vi "1D_Plotter_MATLAB.vi"(1 "Job Directory":path) -> (2 "Saved Automatically?":bool, 3 "gnuplotScript":string, 4 "Plot data file":path)   [LabVIEW 2022 SP3]
uses:
  Data plotting/MATLAB/Plot Style.ctl
  gnuplotScriptComponents/minAndMax.ctl
  gnuplotScriptComponents/AutoManualNumber.ctl
  gnuplotScriptComponents/ticsAndGrids.ctl
  gnuplotScriptComponents/tics.ctl
  gnuplotScriptComponents/grids.ctl
  Error bar Type.ctl
  Data plotting/MATLAB/MATLAB_Mode.ctl
  Results_plotter_Global.vi
  Globals/Constants_global.vi
  Data plotting/subVIs/Plot_Values_Global.vi
panel:
  in  "Tab Control":T1(tab)
  in  "Show Save Option?":bool
  in  "Font Size":string="10"
  in  "MainTitleFontSize":string="12"
  in  "Horizontal/Vertical plot ratio":dbl=1.0 min=0.1 max=10.0 format="%.2f"
  in  "Auto":bool=TRUE
  in  "Open in Acrobat":bool=TRUE
  in  "Stl File":u16(ring)
  in  "Location Y limits":string="-2000;2000"
  in  "Location X limits":string="-2000;2000"
  in  "Plot Location?":bool
  in  "Z Limits Auto":bool=TRUE
  in  "Location Z limits":string="-2000;2000"
  in  "Y Limits Auto":bool=TRUE
  in  "X Limits Auto":bool=TRUE
  in  "Only Show Plots with ALL Series":bool
  in  "nRows":u8=3 min=1
  in  "nCols":u8=3 min=1
  in  "Swop Series and Plots":bool
  in  "Legend Title":string
  out "Number of Figures":i32
  in  "View Angle":string="-20;39"
  in  "lRefArrowSize":string="2"
  in  "lRefArrowColor":string="k"
  in  "lRefArrowComponents":string="300;0;0"
  in  "lRefArrowBaseCoord":string="0;0;0"
  in  "lRefPointSize":string="20"
  in  "lRefPointColor":string="y"
  in  "lRefPointCoord":string="0;0;0"
  in  "fAxisLabelYright":string
  out "Output file":path
  out "Saved Files":path[](array[path])
  in  "Reduce Individual Plot Title Lengths if too long":bool=TRUE
  in  "Show Channels with range of Values?":bool
  in  "ManualPlotTitles":string[](array[string])
  in  "Individual Plot Titles":bool=TRUE
  in  "Page Title Pre Block":string
  in  "Page Title Post Block":string
  in  "Values to include in Page Title":i32[](listbox)
  out "Final Title":string
  out "Plot Titles":string[](array[string])
  in  "Plot Legends Manual":string[](array[string])
  in  "Plotstyles":T2[](array[typedef])=[{"Color"="r", "LStyle"="solid", "LWidth"="0.5", "Marker"="o", "Marker size"="4.0", "Fit?"=FALSE, "Right Y?"=FALSE}, {"Color"="g", "LStyle"="solid", "LWidth"="0.5", "Marker"="+", "Marker size"="4.0", "Fit?"=FALSE, "Right Y?"=FALSE}, {"Color"="b", "LStyle"="solid", "LWidth"="0.5", "Marker"="*", "Marker size"="4.0", "Fit?"=FALSE, "Right Y?"=FALSE}, {"Color"="k", "LStyle"="solid", "LWidth"="0.5", "Marker"=".", "Marker size"="4.0", "Fit?"=FALSE, "Right Y?"=FALSE}, {"Color"="c", "LStyle"="solid", "LWidth"="0.5", "Marker"="x", "Marker size"="4.0", "Fit?"=FALSE, "Right Y?"=FALSE}, {"Color"="m", "LStyle"="solid", "LWidth"="0.5", "Marker"="s", "Marker size"="4.0", "Fit?"=FALSE, "Right Y?"=FALSE}, {"Color"="y", "LStyle"="solid", "LWidth"="0.5", "Marker"="d", "Marker size"="4.0", "Fit?"=FALSE, "Right Y?"=FALSE}, {"Color"="r", "LStyle"="--", "LWidth"="0.5", "Marker"="^", "Marker size"="4.0", "Fit?"=FALSE, "Right Y?"=FALSE}, {"Color"="g", "LStyle"="--", "LWidth"="0.5", "Marker"="v", "Marker size"="4.0", "Fit?"=FALSE, "Right Y?"=FALSE}, {"Color"="b", "LStyle"="--", "LWidth"="0.5", "Marker"="p", "Marker size"="4.0", "Fit?"=FALSE, "Right Y?"=FALSE}, {"Color"="k", "LStyle"="--", "LWidth"="0.5", "Marker"="h", "Marker size"="4.0", "Fit?"=FALSE, "Right Y?"=FALSE}, {"Color"="c", "LStyle"="--", "LWidth"="0.5", "Marker"="x", "Marker size"="4.0", "Fit?"=FALSE, "Right Y?"=FALSE}, {"Color"="m", "LStyle"="--", "LWidth"="0.5", "Marker"=">", "Marker size"="4.0", "Fit?"=FALSE, "Right Y?"=FALSE}] caption="Plot Style"
  out "Plot Legends Auto":string[](array[string])
  out "No of Series supplied":i32
  in  "Plot Legends":bool=TRUE
  in  "Error Bar Type":T3=enum."Standard Error"
  in  "2nd Y Axis":enum8{"Lin", "Log"}(ring)
  in  "Y/R tics And Grids":T4={"tics"={"ticMin"=0.0, "ticStep"=5.0, "ticMax"=0.0, "minorDivsPerMajor"=2, "ticSpacing"=enum."Approx n Tics (rounded)", "ticPosition"=enum."Inside, no mirror"}, "Grids"={"Gridlines"=enum."No grids", "Zeroaxis"=enum."No zero axis"}, "Mapping"=enum."Lin"}
  in  "X/Theta tics And Grids":T4={"tics"={"ticMin"=0.0, "ticStep"=5.0, "ticMax"=0.0, "minorDivsPerMajor"=2, "ticSpacing"=enum."Approx n Tics (rounded)", "ticPosition"=enum."Inside, no mirror"}, "Grids"={"Gridlines"=enum."Major grid", "Zeroaxis"=enum."No zero axis"}, "Mapping"=enum."Lin"}
  in  "PlotType":enum32{"XY", "Time"}(tab)
  in  "yAxisBounds":T7={"Min"={"Auto"=TRUE, "Value"=0.0}, "Max"={"Auto"=TRUE, "Value"=0.0}}
  in  "xAxisBounds":T7={"Min"={"Auto"=TRUE, "Value"=0.0}, "Max"={"Auto"=TRUE, "Value"=0.0}}
  in  "Set bounds using XY Plot \non Results file plotter":bool
  out "Time format?":bool
  in  "Time/Date Format":string(combo)="%I:%M %p\\n%d-%b-%y"
  in  "Select Time Zone":u32(ring)=142 items=["Abbreviation (Time Zone Name)", "A (Alpha Time Zone)", "ACDT (Australian Central Daylight Time  CDT ‚Äì Central Daylight Time CDST ‚Äì Central Daylight Savings Time)", "ACST (Australian Central Standard Time  CST ‚Äì Central Standard Time)", "ACT (Acre Time)", "ACT (Australian Central Time)", "ACWST (Australian Central Western Standard Time)", "ADT (Arabia Daylight Time  AST ‚Äì Arabia Summer Time)", "ADT (Atlantic Daylight Time  ADST ‚Äì Atlantic Daylight Saving Time AST ‚Äì Atlantic Summer Time  HAA ‚Äì Heure Avancv©e de l'Atlantique (French))", "AEDT (Australian Eastern Daylight Time  EDT ‚Äì Eastern Daylight Time EDST ‚Äì Eastern Daylight Saving Time)", "AEST (Australian Eastern Standard Time  EST ‚Äì Eastern Standard Time AET ‚Äì Australian Eastern Time)", "AET (Australian Eastern Time)", "AFT (Afghanistan Time)", "AKDT (Alaska Daylight Time  ADST ‚Äì Alaska Daylight Saving Time)", "AKST (Alaska Standard Time  AT ‚Äì Alaska Time)", "ALMT (Alma-Ata Time)", "AMST (Amazon Summer Time)", "AMST (Armenia Summer Time  AMDT ‚Äì Armenia Daylight Time)", "AMT (Amazon Time)", "AMT (Armenia Time)", "ANAST (Anadyr Summer Time)", "ANAT (Anadyr Time)", "AQTT (Aqtobe Time)", "ART (Argentina Time)", "AST (Arabia Standard Time  AST ‚Äì Arabic Standard Time AST ‚Äì Al Manamah Standard Time)", "AST (Atlantic Standard Time  AT ‚Äì Atlantic Time  AST ‚Äì Tiempo Estv°ndar del Atlv°ntico (Spanish) HNA ‚Äì Heure Normale de l'Atlantique (French))", "AT (Atlantic Time)", "AWDT (Australian Western Daylight Time  WDT ‚Äì Western Daylight Time WST ‚Äì Western Summer Time)", "AWST (Australian Western Standard Time  WST ‚Äì Western Standard Time WAT ‚Äì Western Australia Time)", "AZOST (Azores Summer Time  AZODT ‚Äì Azores Daylight Time)", "AZOT (Azores Time  AZOST ‚Äì Azores Standard Time)", "AZST (Azerbaijan Summer Time)", "AZT (Azerbaijan Time)", "AoE (Anywhere on Earth)", "B (Bravo Time Zone)", "BNT (Brunei Darussalam Time  BDT ‚Äì Brunei Time)", "BOT (Bolivia Time)", "BRST (Brasv?lia Summer Time  BST ‚Äì Brazil Summer Time BST ‚Äì Brazilian Summer Time)", "BRT (Brasv?lia Time  BT ‚Äì Brazil Time BT ‚Äì Brazilian Time)", "BST (Bangladesh Standard Time)", "BST (Bougainville Standard Time)", "BST (British Summer Time  BDT ‚Äì British Daylight Time BDST ‚Äì British Daylight Saving Time)", "BTT (Bhutan Time)", "C (Charlie Time Zone)", "CAST (Casey Time)", "CAT (Central Africa Time)", "CCT (Cocos Islands Time)", "CDT (Central Daylight Time  CDST ‚Äì Central Daylight Saving Time NACDT ‚Äì North American Central Daylight Time  HAC ‚Äì Heure Avancv©e du Centre (French))", "CDT (Cuba Daylight Time)", "CEST (Central European Summer Time  CEDT ‚Äì Central European Daylight Time ECST ‚Äì European Central Summer Time  MESZ ‚Äì Mitteleuropv§ische Sommerzeit (German))", "CET (Central European Time  ECT ‚Äì European Central Time CET ‚Äì Central Europe Time  MEZ ‚Äì Mitteleuropv§ische Zeit (German))", "CHADT (Chatham Island Daylight Time  CDT ‚Äì Chatham Daylight Time)", "CHAST (Chatham Island Standard Time)", "CHOST (Choibalsan Summer Time  CHODT ‚Äì Choibalsan Daylight Time CHODST ‚Äì Choibalsan Daylight Saving Time)", "CHOST (Choibalsan Summer Time)", "CHOT (Choibalsan Time)", "CHUT (Chuuk Time)", "CIDST (Cayman Islands Daylight Saving Time)", "CIST (Cayman Islands Standard Time  CIT ‚Äì Cayman Islands Time)", "CKT (Cook Island Time)", "CLST (Chile Summer Time  CLDT ‚Äì Chile Daylight Time)", "CLT (Chile Standard Time  CT ‚Äì Chile Time CLST ‚Äì Chile Standard Time)", "COT (Colombia Time)", "CST (Central Standard Time  CT ‚Äì Central Time NACST ‚Äì North American Central Standard Time  CST ‚Äì Tiempo Central Estv°ndar (Spanish) HNC ‚Äì Heure Normale du Centre (French))", "CST (China Standard Time)", "CST (Cuba Standard Time)", "CT (Central Time)", "CVT (Cape Verde Time)", "CXT (Christmas Island Time)", "ChST (Chamorro Standard Time  GST ‚Äì Guam Standard Time)", "D (Delta Time Zone)", "DAVT (Davis Time)", "DDUT (Dumont-d'Urville Time)", "E (Echo Time Zone)", "EASST (Easter Island Summer Time  EADT ‚Äì Easter Island Daylight Time)", "EAST (Easter Island Standard Time)", "EAT (Eastern Africa Time  EAT ‚Äì East Africa Time)", "ECT (Ecuador Time)", "EDT (Eastern Daylight Time  EDST ‚Äì Eastern Daylight Savings Time NAEDT ‚Äì North American Eastern Daylight Time  HAE ‚Äì Heure Avancv©e de l'Est (French) EDT ‚Äì Tiempo de verano del Este (Spanish))", "EEST (Eastern European Summer Time  EEDT ‚Äì Eastern European Daylight Time  OESZ ‚Äì Osteuropv§ische Sommerzeit (German))", "EET (Eastern European Time  OEZ ‚Äì Osteuropv§ische Zeit (German))", "EGST (Eastern Greenland Summer Time  EGST ‚Äì East Greenland Summer Time)", "EGT (East Greenland Time  EGT ‚Äì Eastern Greenland Time)", "EST (Eastern Standard Time  ET ‚Äì Eastern Time  NAEST ‚Äì North American Eastern Standard Time  ET ‚Äì Tiempo del Este (Spanish) HNE ‚Äì Heure Normale de l'Est (French))", "ET (Eastern Time)", "F (Foxtrot Time Zone)", "FET (Further-Eastern European Time)", "FJST (Fiji Summer Time  FJDT ‚Äì Fiji Daylight Time)", "FJT (Fiji Time)", "FKST (Falkland Islands Summer Time  FKDT ‚Äì Falkland Island Daylight Time)", "FKT (Falkland Island Time  FKST ‚Äì Falkland Island Standard Time)", "FNT (Fernando de Noronha Time)", "G (Golf Time Zone)", "GALT (Galapagos Time)", "GAMT (Gambier Time  GAMT ‚Äì Gambier Islands Time)", "GET (Georgia Standard Time)", "GFT (French Guiana Time)", "GILT (Gilbert Island Time)", "GMT (Greenwich Mean Time  \"‚Äì Coordinated Universal Time GT ‚Äì Greenwich Time)", "GST (Gulf Standard Time)", "GST (South Georgia Time)", "GYT (Guyana Time)", "H (Hotel Time Zone)", "HADT (Hawaii-Aleutian Daylight Time  HDT ‚Äì Hawaii Daylight Time)", "HAST (Hawaii-Aleutian Standard Time  HST ‚Äì Hawaii Standard Time)", "HKT (Hong Kong Time)", "HOVST (Hovd Summer Time  HOVDT ‚Äì Hovd Daylight Time HOVDST ‚Äì Hovd Daylight Saving Time)", "HOVST (Hovd Summer Time)", "HOVT (Hovd Time)", "I (India Time Zone)", "ICT (Indochina Time)", "IDT (Israel Daylight Time)", "IOT (Indian Chagos Time)", "IRDT (Iran Daylight Time  IRST ‚Äì Iran Summer Time IDT ‚Äì Iran Daylight Time)", "IRKST (Irkutsk Summer Time)", "IRKT (Irkutsk Time)", "IRST (Iran Standard Time  IT ‚Äì Iran Time)", "IST (India Standard Time  IT ‚Äì India Time IST ‚Äì Indian Standard Time)", "IST (Irish Standard Time  IST ‚Äì Irish Summer Time)", "IST (Israel Standard Time)", "JST (Japan Standard Time)", "K (Kilo Time Zone)", "KGT (Kyrgyzstan Time)", "KOST (Kosrae Time)", "KRAST (Krasnoyarsk Summer Time)", "KRAT (Krasnoyarsk Time)", "KST (Korea Standard Time  KST ‚Äì Korean Standard Time KT ‚Äì Korea Time)", "KUYT (Kuybyshev Time  SAMST ‚Äì Samara Summer Time)", "L (Lima Time Zone)", "LHDT (Lord Howe Daylight Time)", "LHST (Lord Howe Standard Time)", "LINT (Line Islands Time)", "M (Mike Time Zone)", "MAGST (Magadan Summer Time  MAGST ‚Äì Magadan Island Summer Time)", "MAGT (Magadan Time  MAGT ‚Äì Magadan Island Time)", "MART (Marquesas Time)", "MAWT (Mawson Time)", "MDT (Mountain Daylight Time  MDST ‚Äì Mountain Daylight Saving Time NAMDT ‚Äì North American Mountain Daylight Time  HAR ‚Äì Heure Avancv©e des Rocheuses (French))", "MHT (Marshall Islands Time)", "MMT (Myanmar Time)", "MSD (Moscow Daylight Time  Moscow Summer Time)", "MSK (Moscow Standard Time  MCK ‚Äì Moscow Time)", "MST (Mountain Standard Time  MT ‚Äì Mountain Time NAMST ‚Äì North American Mountain Standard Time  HNR ‚Äì Heure Normale des Rocheuses (French))", "MT (Mountain Time)", "MUT (Mauritius Time)", "MVT (Maldives Time)", "MYT (Malaysia Time  MST ‚Äì Malaysian Standard Time)", "N (November Time Zone)", "NCT (New Caledonia Time)", "NDT (Newfoundland Daylight Time  HAT ‚Äì Heure Avancv©e de Terre-Neuve (French))", "NFT (Norfolk Time  NFT ‚Äì Norfolk Island Time)", "NOVST (Novosibirsk Summer Time  OMSST ‚Äì Omsk Summer Time)", "NOVT (Novosibirsk Time  OMST ‚Äì Omsk Standard Time)", "NPT (Nepal Time)", "NRT (Nauru Time)", "NST (Newfoundland Standard Time  HNT ‚Äì Heure Normale de Terre-Neuve (French))", "NUT (Niue Time)", "NZDT (New Zealand Daylight Time)", "NZST (New Zealand Standard Time)", "O (Oscar Time Zone)", "OMSST (Omsk Summer Time  NOVST ‚Äì Novosibirsk Summer Time)", "OMST (Omsk Standard Time  OMST ‚Äì Omsk Time NOVT ‚Äì Novosibirsk Time)", "ORAT (Oral Time)", "P (Papa Time Zone)", "PDT (Pacific Daylight Time  PDST ‚Äì Pacific Daylight Saving Time NAPDT ‚Äì North American Pacific Daylight Time  HAP ‚Äì Heure Avancv©e du Pacifique (French))", "PET (Peru Time)", "PETST (Kamchatka Summer Time)", "PETT (Kamchatka Time  PETT ‚Äì Petropavlovsk-Kamchatski Time)", "PGT (Papua New Guinea Time)", "PHOT (Phoenix Island Time)", "PHT (Philippine Time  PST ‚Äì Philippine Standard Time)", "PKT (Pakistan Standard Time  PKT ‚Äì Pakistan Time)", "PMDT (Pierre & Miquelon Daylight Time)", "PMST (Pierre & Miquelon Standard Time)", "PONT (Pohnpei Standard Time)", "PST (Pacific Standard Time  PT ‚Äì Pacific Time NAPST ‚Äì North American Pacific Standard Time  PT ‚Äì Tiempo del Pacv?fico (Spanish) HNP ‚Äì Heure Normale du Pacifique (French))", "PST (Pitcairn Standard Time)", "PT (Pacific Time)", "PWT (Palau Time)", "PYST (Paraguay Summer Time)", "PYT (Paraguay Time)", "PYT (Pyongyang Time  PYST ‚Äì Pyongyang Standard Time)", "PYT (Pyongyang Time)", "Q (Quebec Time Zone)", "QYZT (Qyzylorda Time)", "R (Romeo Time Zone)", "RET (Reunion Time)", "ROTT (Rothera Time)", "S (Sierra Time Zone)", "SAKT (Sakhalin Time)", "SAMT (Samara Time  SAMT ‚Äì Samara Standard Time)", "SAST (South Africa Standard Time  SAST ‚Äì South African Standard Time)", "SBT (Solomon Islands Time  SBT ‚Äì Solomon Island Time)", "SCT (Seychelles Time)", "SGT (Singapore Time  SST ‚Äì Singapore Standard Time)", "SRET (Srednekolymsk Time)", "SRT (Suriname Time)", "SST (Samoa Standard Time)", "SYOT (Syowa Time)", "T (Tango Time Zone)", "TAHT (Tahiti Time)", "TFT (French Southern and Antarctic Time  KIT ‚Äì Kerguelen (Islands) Time)", "TJT (Tajikistan Time)", "TKT (Tokelau Time)", "TLT (East Timor Time)", "TMT (Turkmenistan Time)", "TOT (Tonga Time)", "TVT (Tuvalu Time)", "U (Uniform Time Zone)", "ULAST (Ulaanbaatar Summer Time  ULAST ‚Äì Ulan Bator Summer Time)", "ULAST (Ulaanbaatar Summer Time)", "ULAT (Ulaanbaatar Time  ULAT ‚Äì Ulan Bator Time)", "ULAT (Ulaanbaatar Time)", "UTC (Coordinated Universal Time)", "UYST (Uruguay Summer Time)", "UYT (Uruguay Time)", "UZT (Uzbekistan Time)", "V (Victor Time Zone)", "VET (Venezuelan Standard Time  HLV ‚Äì Hora Legal de Venezuela (Spanish))", "VLAST (Vladivostok Summer Time)", "VLAT (Vladivostok Time)", "VOST (Vostok Time)", "VUT (Vanuatu Time  EFATE ‚Äì Efate Time)", "W (Whiskey Time Zone)", "WAKT (Wake Time)", "WARST (Western Argentine Summer Time)", "WAST (West Africa Summer Time)", "WAT (West Africa Time)", "WEST (Western European Summer Time  WEDT ‚Äì Western European Daylight Time  WESZ ‚Äì Westeuropv§ische Sommerzeit (German))", "WET (Western European Time  GMT ‚Äì Greenwich Mean Time  WEZ ‚Äì Westeuropv§ische Zeit (German))", "WFT (Wallis and Futuna Time)", "WGST (Western Greenland Summer Time  WGST ‚Äì West Greenland Summer Time)", "WGT (West Greenland Time  WGT ‚Äì Western Greenland Time)", "WIB (Western Indonesian Time  WIB ‚Äì Waktu Indonesia Barat)", "WIT (Eastern Indonesian Time  WIT ‚Äì Waktu Indonesia Timur)", "WITA (Central Indonesian Time  WITA ‚Äì Waktu Indonesia Tengah)", "WST (West Samoa Time  ST ‚Äì Samoa Time)", "WST (Western Sahara Summer Time)", "WT (Western Sahara Standard Time  WT ‚Äì Western Sahara Time)", "X (X-ray Time Zone)", "Y (Yankee Time Zone)", "YAKST (Yakutsk Summer Time)", "YAKT (Yakutsk Time)", "YAPT (Yap Time)", "YEKST (Yekaterinburg Summer Time)", "YEKT (Yekaterinburg Time)", "Z (Zulu Time Zone)"]
  out "Time Format String":string="%I:%M %p\\n%d-%b-%y"
  out "Formatted date/time string":string="05:00 PM\\n21-Jan-16"
  out "TZ Shift (hrs)":string="UTC-7.00"
  out "ILocationRotations":string
  out "AuditTrail":string[](array[string])
  out "Desired Legends":string[][](array[string])
  out "Table":string[][](table)
  in  "Put Coeff\nin Results file":bool
  in  "Fit type":T9(ring)=enum."Gauss Vert"
  out "Coeff":string[][](array[string])
  out "subarray":string[](array[string])
  out "Plot Array":i32[][](array[numeric])
  in  "stl file String":string="MAGIC_London_Southbank_0_deg.stl"
  out "Array":path[](array[path])
  out "stl Limits":sgl[][](array[numeric])
  out "Legend Location":string
  out "No of Series":i32
  out "Dont show axis label":bool
  out "Duplicate Plot":bool
  out "Multi_Plot":bool
  out "Y labels":bool[](array[boolean])
  out "X Labels":bool[](array[boolean])
  out "Plot Array initial":i32[][](array[numeric])
  out "Plot Folder":string[](array[string])
  out "Max Min array":dbl[][][](array[numeric])
  out "Error Bars":bool[][](array[boolean])
  out "Y Names":string[](array[string])
  out "X Names":string[](array[string])
  out "X Pos":dbl[](array[numeric])
  out "Y Pos":dbl[](array[numeric])
  out "Z Pos":dbl[](array[numeric])
  # "Rows/ Columns/ Series from: controls not wired- just a thought for explicit control of what goes where...?"
  # "Location Plot"
  # "Overall Page Title"
  # "There are as many graphs as there are titles (from Selector 2)...."
  # "Plot Styles"
  # "Each graph contains plots from Selector 1..."
  # "X"
  # "Y"
  # "Shows the numbered line colours and point styles available- well it would, if it didn't disappear every time I update from the repository..!"
  # "You have to save the plot for this to work"
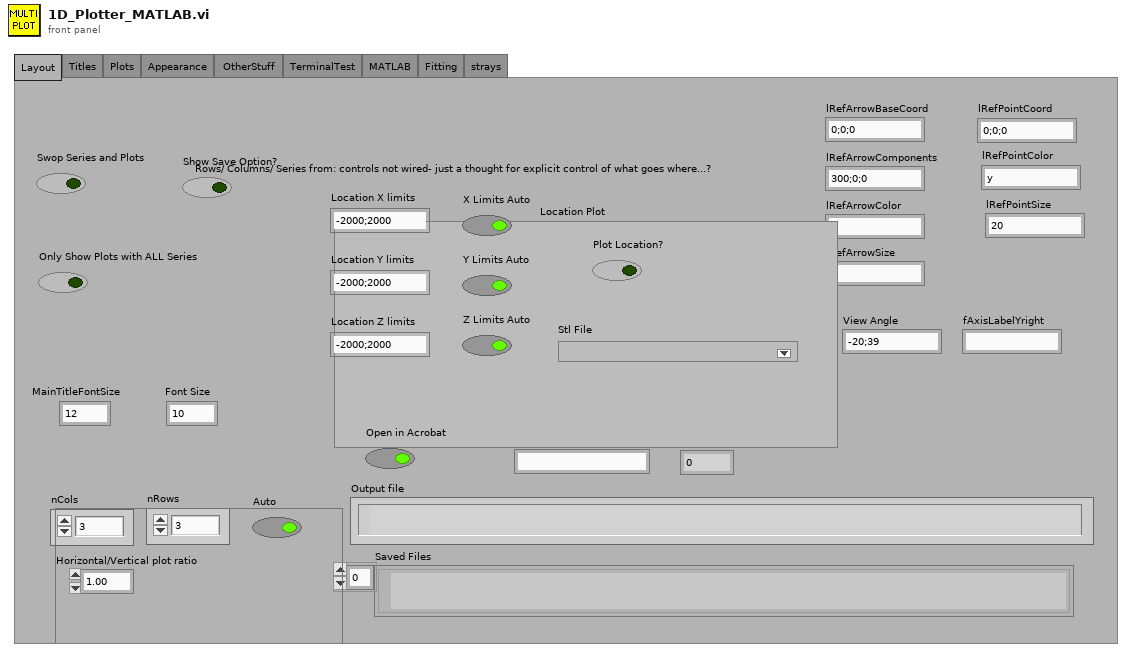
[diagram p1: front panel]
types:
  T1 = enum32{"Layout", "Titles", "Plots", "Appearance", "OtherStuff ", "TerminalTest", "MATLAB", "Fitting", "strays"}
  T2 = typedef "Plot Style.ctl" = cluster{"Color":string, "LStyle":string, "LWidth":string, "Marker":string, "Marker size":string, "Fit?":bool, "Right Y?":bool}
  T3 = typedef "Error bar Type.ctl" = enum16{"None", "Standard Error", "Separate upper and lower"}
  T4 = typedef "ticsAndGrids.ctl" = cluster{"tics":T5, "Grids":T6, "Mapping":enum8{"Lin", "Log"}}
  T5 = typedef "tics.ctl" = cluster{"ticMin":dbl, "ticStep":dbl, "ticMax":dbl, "minorDivsPerMajor":i32, "ticSpacing":enum16{"Auto Tics", "Fixed spacing", "Fixed Minimum and Spacing", "Start, Spacing and Maximum", "Approx n Tics (rounded)"}, "ticPosition":enum16{"Inside, no mirror", "Inside, mirrored", "Outside, no mirror", "Outside, mirrored", "Invisible"}}
  T6 = typedef "grids.ctl" = cluster{"Gridlines":enum16{"No grids", "Major grid", "Minor grid", "Major and Minor"}, "Zeroaxis":enum16{"No zero axis", "Show zero axis"}}
  T7 = typedef "minAndMax.ctl" = cluster{"Min":T8, "Max":T8}
  T8 = typedef "AutoManualNumber.ctl" = cluster{"Auto":bool, "Value":dbl}
  T9 = enum16{"None", "Linear", "2nd Poly", "3rd Poly", "4th Poly", "Gauss Lat", "Gauss Vert", "Guass glc"}
  T10 = enum16{"No grids", "Major grid", "Minor grid", "Major and Minor"}
  T11 = typedef "MATLAB_Mode.ctl" = enum16{"1D Plotter", "2D Plotter", "LP Plotter", "7HP UVW"}
  T12 = typedef "RFP_Plot_Metadata.ctl" = cluster{"Row Number":i32[], "Error Bars":T13, "X Label":string, "Y Label":string, "Blanks NaNs":i32[]}
  T13 = typedef "Error_bars_index.ctl" = cluster{"Upper":i32, "Lower":i32, "St Error":i32}
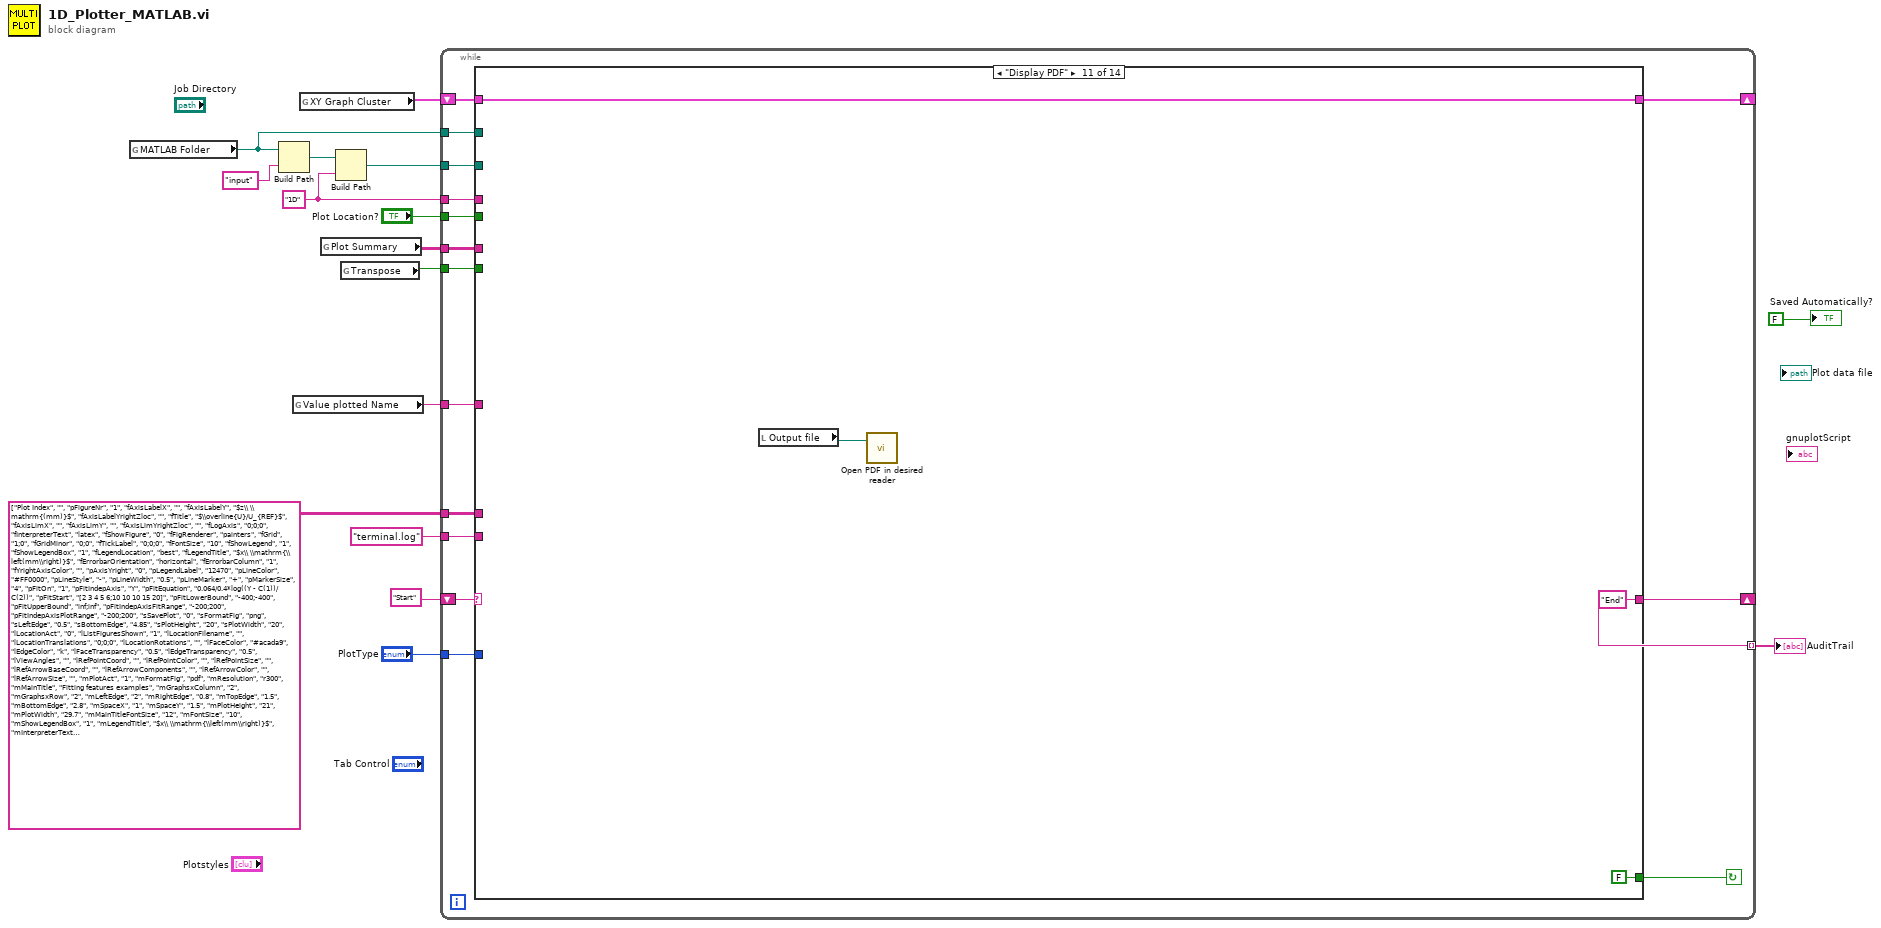
[diagram p0: block diagram]
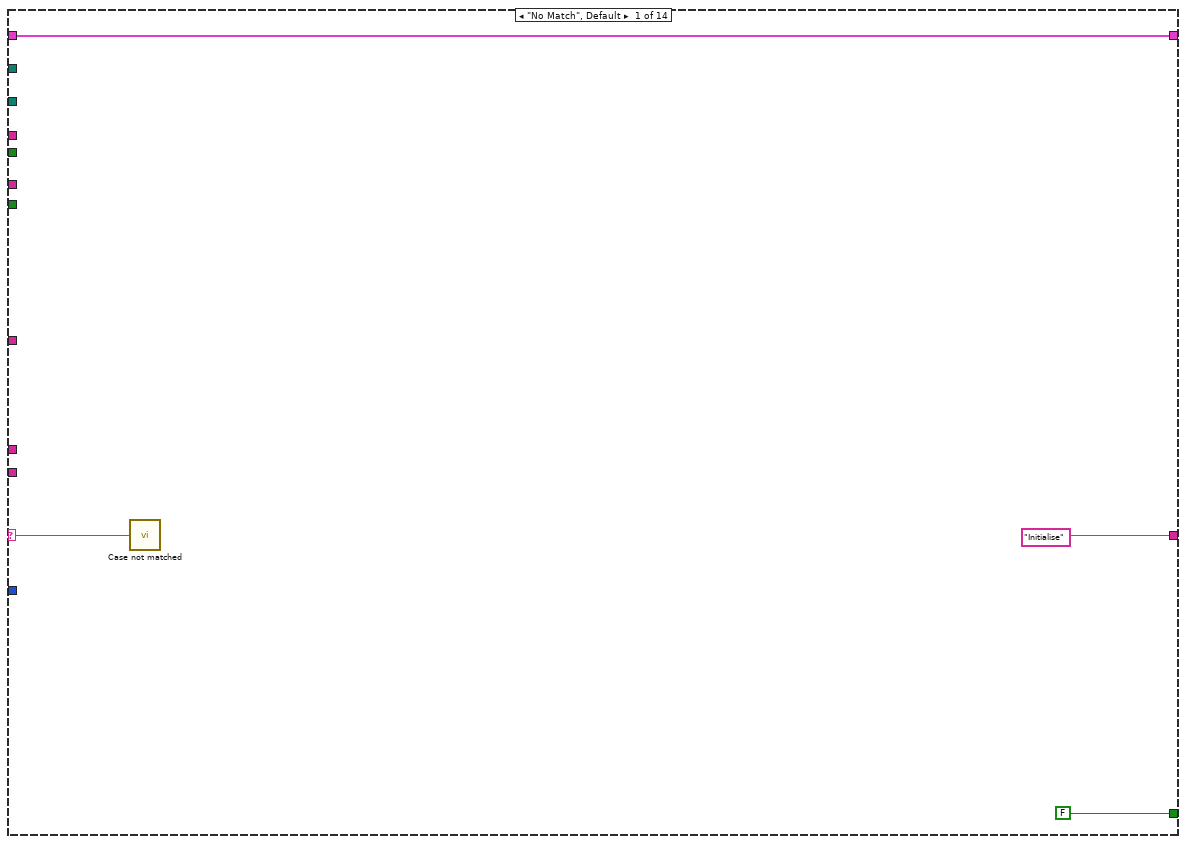
[diagram p2: hidden frame]
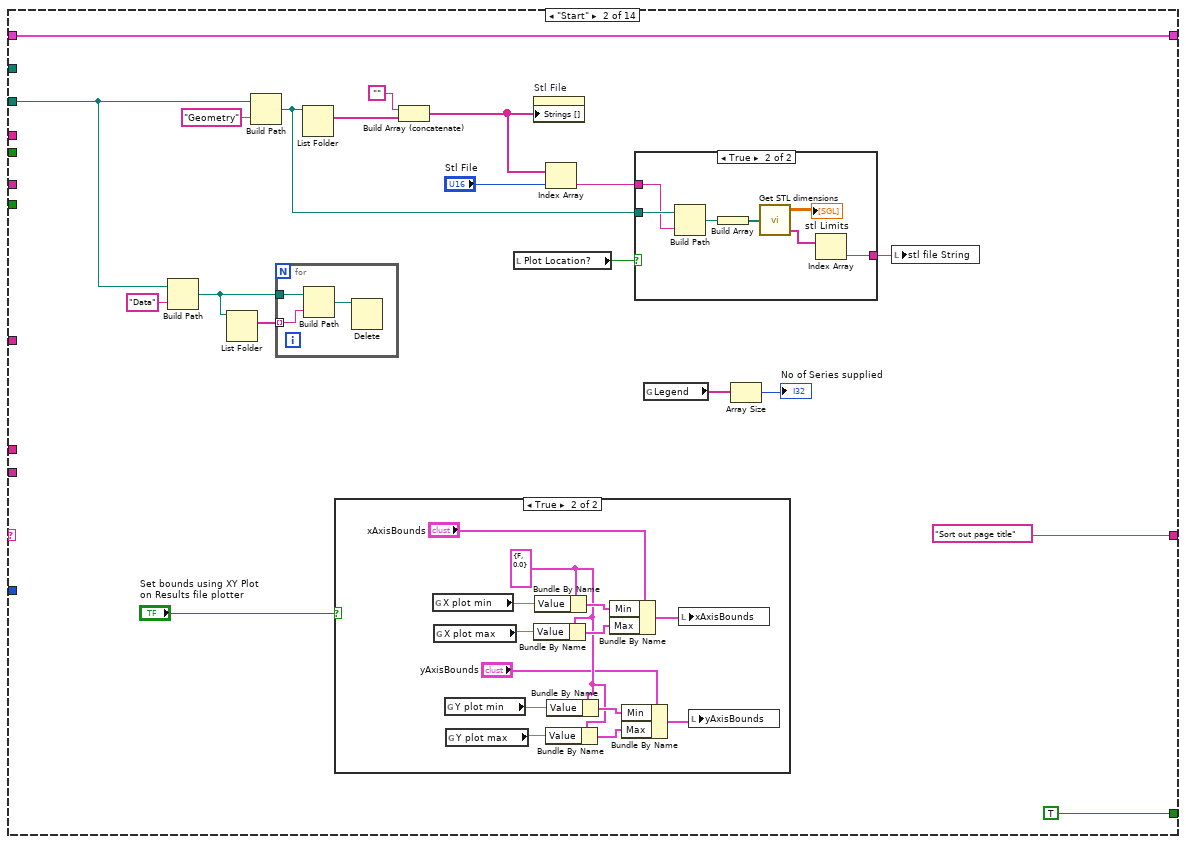
[diagram p3: hidden frame]
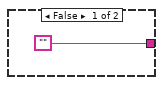
[diagram p4: hidden frame]
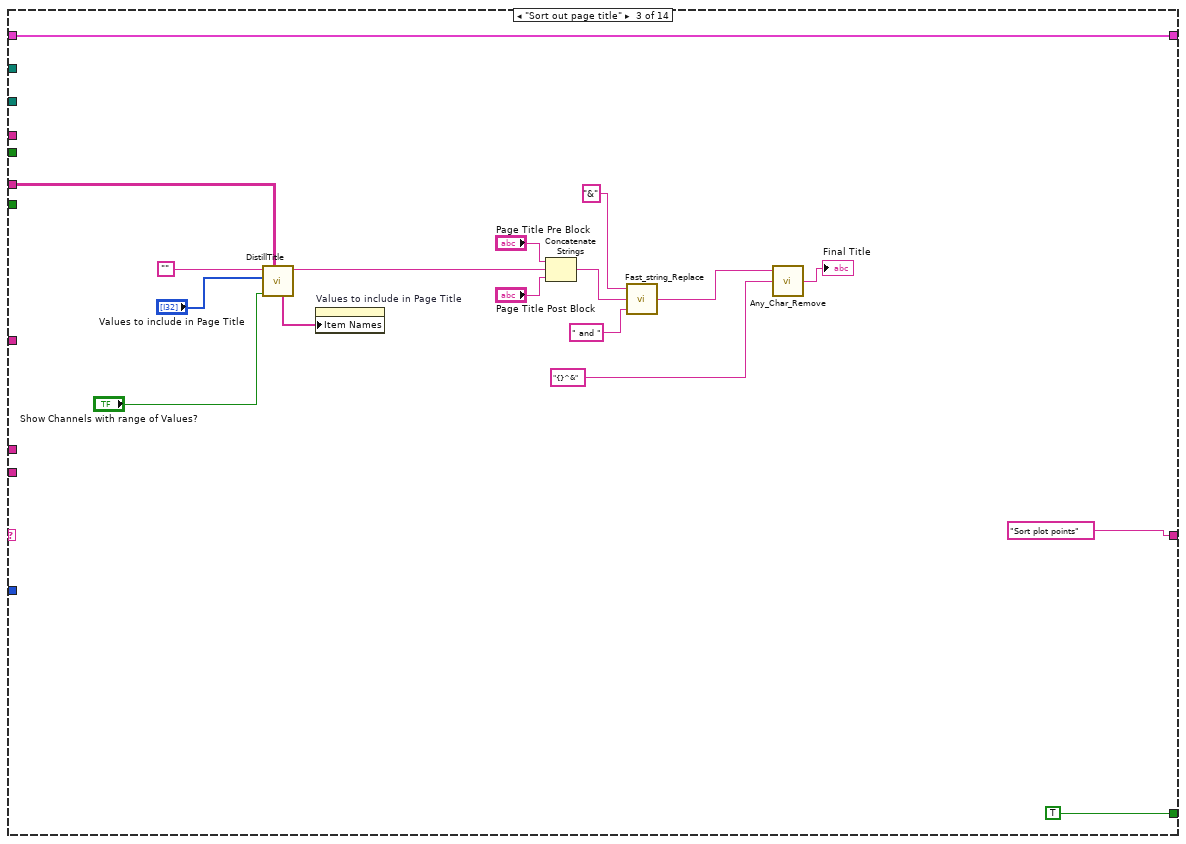
[diagram p6: hidden frame]
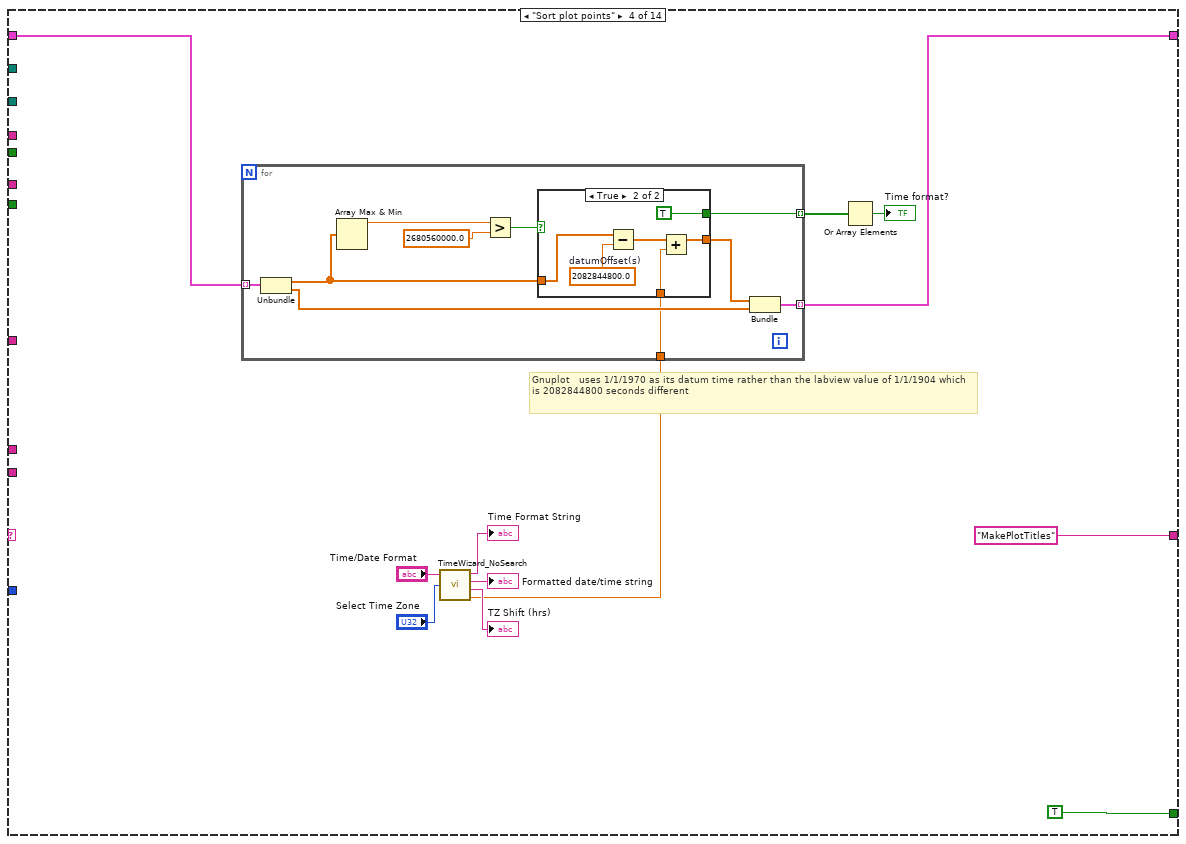
[diagram p7: hidden frame]
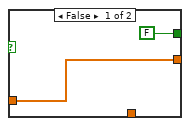
[diagram p8: hidden frame]
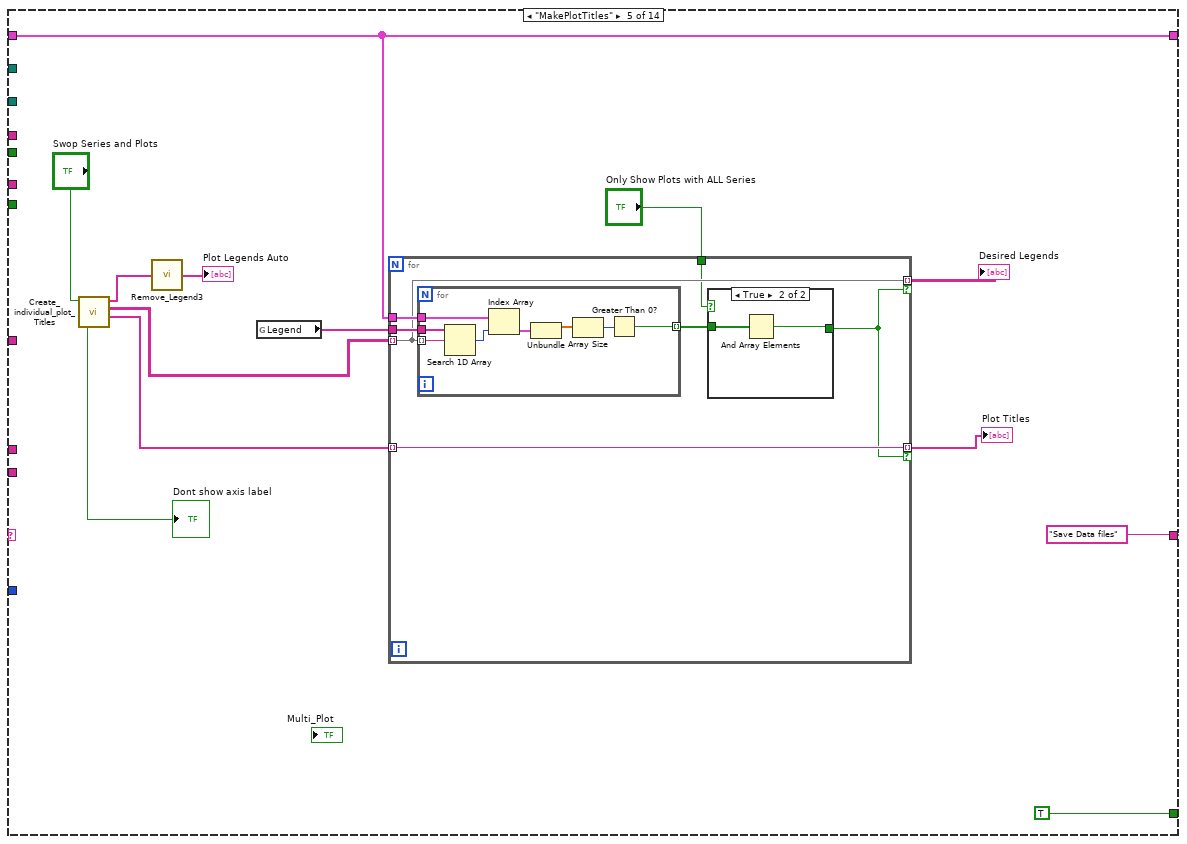
[diagram p9: hidden frame]
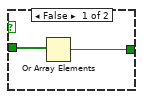
[diagram p10: hidden frame]
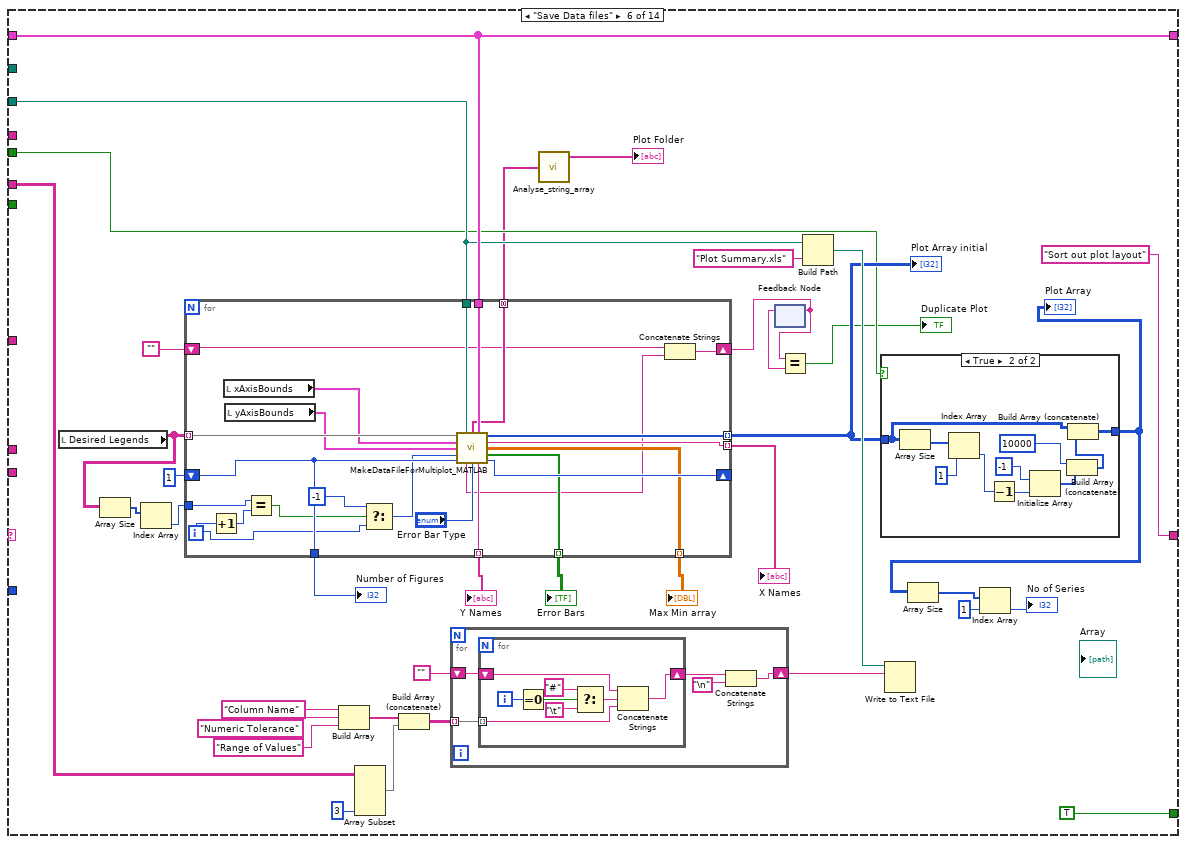
[diagram p11: hidden frame]
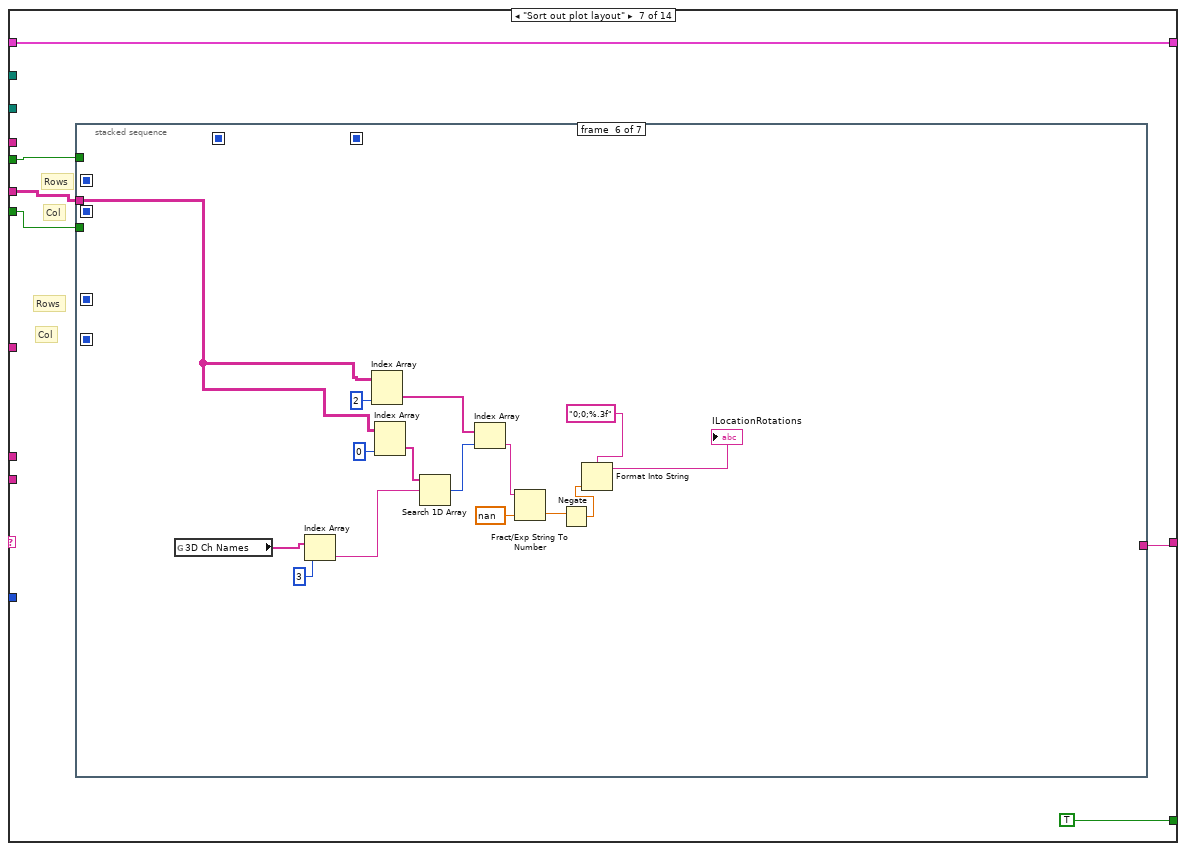
[diagram p13: hidden frame]
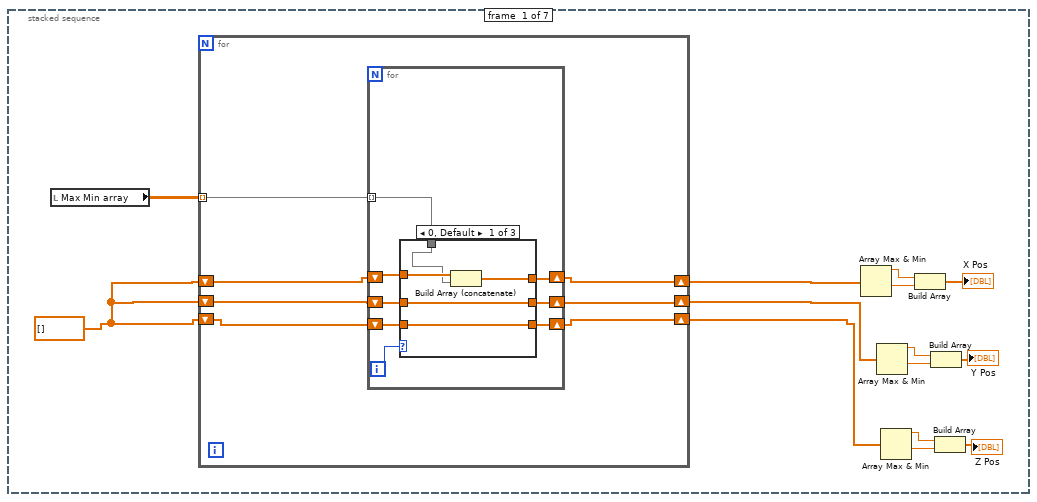
[diagram p14: hidden frame]
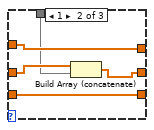
[diagram p15: hidden frame]
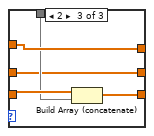
[diagram p16: hidden frame]
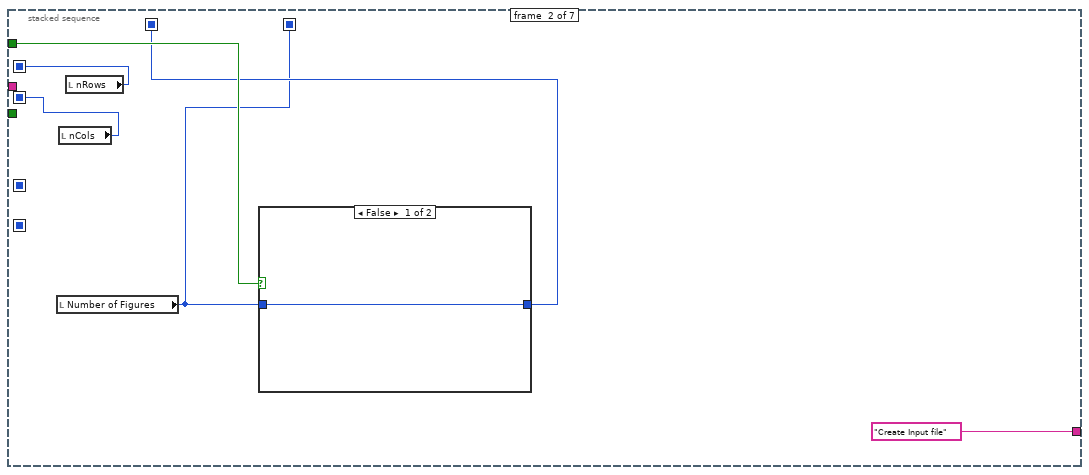
[diagram p17: hidden frame]
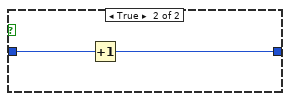
[diagram p18: hidden frame]
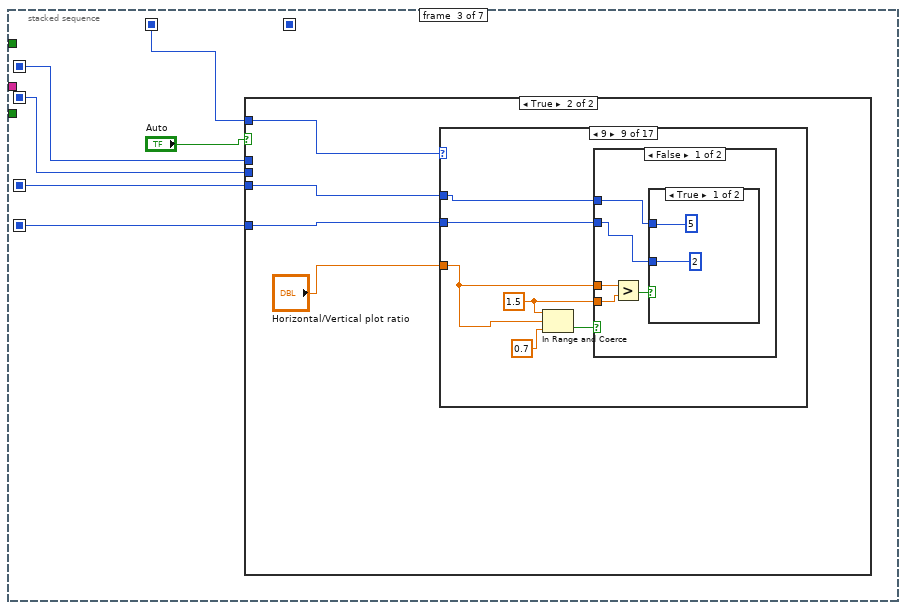
[diagram p19: hidden frame]
diagram:
  w1 = "1D" ("name or relative path")
  n1 = global read "Constants_global.vi" "MATLAB Folder"() -> (w2:path)
  n2 = Build Path(base path=w2, name or relative path="input") -> (appended path=w8:path)
  n3 = global read "Results_plotter_Global.vi" "Value plotted Name"() -> (w14:string)
  n4 = global read "Plot_Values_Global.vi" "XY Graph Cluster"() -> (w3:cluster{dbl[], dbl[]}[])
  n5 = global read "Results_plotter_Global.vi" "Plot Summary"() -> (w15:string[][])
  n6 = Build Path(base path=w8, name or relative path=w1) -> (appended path=w7:path)
  n7 = global read "Results_plotter_Global.vi" "Transpose"() -> (w4:bool)
  n8 = while {
    shift-left: "Start" -> [w30]
    shift-right: [w23] -> _
    tunnel: w15 -> [w29]
    tunnel: w14 -> [w28]
    shift-right: [w26] -> _
    shift-left: w3 -> [w27]
    tunnel: "terminal.log" -> [w25]
    tunnel: w4 -> [w24]
    tunnel: [w23] -> w11 mode=indexing
    tunnel: "PlotType" -> [w22]
    tunnel: w7 -> [w21]
    tunnel: "Plot Location?" -> [w20]
    tunnel: string[][] [["Plot Index", ""], ["pFigureNr", "1"], ["fAxisLabelX", ""], ["fAxisLabelY", "$z\\ \\mathrm{(mm)}$"], ["fAxisLabelYrightZloc", ""], ["fTitle", "$\\overline{U}/U_{REF}$"], ["fAxisLimX", ""], ["fAxisLimY", ""], ["fAxisLimYrightZloc", ""], ["fLogAxis", "0;0;0"], ["fInterpreterText", "latex"], ["fShowFigure", "0"], ["fFigRenderer", "painters"], ["fGrid", "1;0"], ["fGridMinor", "0;0"], ["fTickLabel", "0;0;0"], ["fFontSize", "10"], ["fShowLegend", "1"], ["fShowLegendBox", "1"], ["fLegendLocation", "best"], ["fLegendTitle", "$x\\ \\mathrm{\\left(mm\\right)}$"], ["fErrorbarOrientation", "horizontal"], ["fErrorbarColumn", "1"], ["fYrightAxisColor", ""], ["pAxisYright", "0"], ["pLegendLabel", "12470"], ["pLineColor", "#FF0000"], ["pLineStyle", "-"], ["pLineWidth", "0.5"], ["pLineMarker", "+"], ["pMarkerSize", "4"], ["pFitOn", "1"], ["pFitIndepAxis", "Y"], ["pFitEquation", "0.064/0.4*log((Y - C(1))/C(2))"], ["pFitStart", "[2 3 4 5 6;10 10 10 15 20]"], ["pFitLowerBound", "-400;-400"], ["pFitUpperBound", "inf;inf"], ["pFitIndepAxisFitRange", "-200;200"], ["pFitIndepAxisPlotRange", "-200;200"], ["sSavePlot", "0"], ["sFormatFig", "png"], ["sLeftEdge", "0.5"], ["sBottomEdge", "4.85"], ["sPlotHeight", "20"], ["sPlotWidth", "20"], ["lLocationAct", "0"], ["lListFiguresShown", "1"], ["lLocationFilename", ""], ["lLocationTranslations", "0;0;0"], ["lLocationRotations", ""], ["lFaceColor", "#acada9"], ["lEdgeColor", "k"], ["lFaceTransparency", "0.5"], ["lEdgeTransparency", "0.5"], ["lViewAngles", ""], ["lRefPointCoord", ""], ["lRefPointColor", ""], ["lRefPointSize", ""], ["lRefArrowBaseCoord", ""], ["lRefArrowComponents", ""], ["lRefArrowColor", ""], ["lRefArrowSize", ""], ["mPlotAct", "1"], ["mFormatFig", "pdf"], ["mResolution", "r300"], ["mMainTitle", "Fitting features examples"], ["mGraphsxColumn", "2"], ["mGraphsxRow", "2"], ["mLeftEdge", "2"], ["mRightEdge", "0.8"], ["mTopEdge", "1.5"], ["mBottomEdge", "2.8"], ["mSpaceX", "1"], ["mSpaceY", "1.5"], ["mPlotHeight", "21"], ["mPlotWidth", "29.7"], ["mMainTitleFontSize", "12"], ["mFontSize", "10"], ["mShowLegendBox", "1"], ["mLegendTitle", "$x\\ \\mathrm{\\left(mm\\right)}$"], ["mInterpreterText", "latex"], ["mFigRenderer", "opengl"], ["mLegendLocation", "0.5;0.05"], ["mLegendColumnNr", "1"]] ("subarray") -> [w19]
    tunnel: w2 -> [w18]
    tunnel: w1 -> [w17]
    stop <- w31 continue-if-true
    n9 = case shown="\"Display PDF\"" w30 {
      selector: w30 -> [w32 _ _ _ _ _ _ _ _ _ _ _ _ _]
      tunnel: [FALSE TRUE TRUE ("Top Level") TRUE TRUE ("Top Level") TRUE ("Top Level") TRUE ("Top Level") TRUE ("Top Level") TRUE ("Top Level") w1239 FALSE ("Top Level") w1249 FALSE ("Top Level") FALSE ("Top Level")] -> w31
      tunnel: ["Initialise" "Sort out page title" "Sort plot points" "MakePlotTitles" "Save Data files" "Sort out plot layout" w243 "Save input file" "Run MATLAB Code" ("t") w1233 "End" ("t") "Get Fit Coeff" ("t") "" ("t") "End" ("t")] -> w23
      tunnel: w29 -> [_ _ w89 _ _ w183 w244 w703 _ _ _ _ _ _]
      tunnel: w28 -> [_ _ _ _ _ _ _ _ _ _ _ _ w1278 _]
      tunnel: w27 -> [w33 w52 w95 w105 w130 w194 w247 w700 w1231 w1240 w1248 w1252 w1282 w1415]
      tunnel: [w33 w52 w95 w104 w130 w194 w247 w700 w1231 w1240 w1248 w1252 w1282 w1415] -> w26
      tunnel: w25 -> [_ _ _ _ _ _ _ _ _ _ _ _ _ _]
      tunnel: w24 -> [_ _ _ _ _ _ w242 _ _ _ _ _ _ _]
      tunnel: w22 -> [_ _ _ _ _ _ _ _ _ _ _ _ _ _]
      tunnel: w21 -> [_ w42 _ _ _ w179 _ w699 w1226 _ _ _ _ _]
      tunnel: w20 -> [_ _ _ _ _ w175 w245 _ _ _ _ _ _ _]
      tunnel: w19 -> [_ _ _ _ _ _ _ w708 w1222 _ _ _ w1279 _]
      tunnel: w18 -> [_ _ _ _ _ _ _ _ w1211 _ _ _ _ _]
      tunnel: w17 -> [_ _ _ _ _ _ _ _ w1210 _ _ _ _ _]
      frame "No Match", Default {
        n10 = call "Case not matched.vi"("Case Name not Matched"=w32) -> ()
      }
      frame "Start" {
        n11 = Build Path(base path=w42, name or relative path="Data") -> (appended path=w47:path)
        n12 = List Folder(path=w47) -> (filenames=w49:string[])  [unwired: 3 in, 3 out]
        n13 = Build Path(base path=w42, name or relative path="Geometry") -> (appended path=w39:path)
        n14 = for {
          tunnel: w49 -> [w65] mode=indexing
          tunnel: w47 -> [w64]
          n15 = Build Path(base path=w64, name or relative path=w65) -> (appended path=w63:path)
          n16 = Delete(path (use dialog)=w63) -> ()  [unwired: 4 in, 3 out]
        }
        n17 = List Folder(path=w39) -> (filenames=w45:string[])  [unwired: 3 in, 3 out]
        n18 = case shown="True" "Set bounds using XY Plot \non Results file plotter" {
          frame False {
          }
          frame True {
            w69 = T8 {"Auto"=FALSE, "Value"=0.0} ("Min")
            n19 = global read "Results_plotter_Global.vi" "X plot min"() -> (w74:dbl)
            n20 = global read "Results_plotter_Global.vi" "X plot max"() -> (w75:dbl)
            n21 = global read "Results_plotter_Global.vi" "Y plot min"() -> (w73:dbl)
            n22 = global read "Results_plotter_Global.vi" "Y plot max"() -> (w72:dbl)
            n23 = Bundle By Name(cluster=w69, "Value"=w75) -> (w77:T8)
            n24 = Bundle By Name(cluster=w69, "Value"=w74) -> (w78:T8)
            n25 = Bundle By Name(cluster=w69, "Value"=w72) -> (w71:T8)
            n26 = Bundle By Name(cluster=w69, "Value"=w73) -> (w70:T8)
            n27 = Bundle By Name(cluster="xAxisBounds", "Min"=w78, "Max"=w77) -> (w76:T7)
            n28 = Bundle By Name(cluster="yAxisBounds", "Min"=w70, "Max"=w71) -> (w68:T7)
            n29 = local write "xAxisBounds"(w76) -> ()
            n30 = local write "yAxisBounds"(w68) -> ()
          }
        }
        n31 = Build Array (concatenate)("", w45) -> (w40:string[])
        n32 = local read "Plot Location?"() -> (w38:bool)
        n33 = property on="Stl File" class="Ring (strict)"("Strings []"=w40) -> ()  [unwired: 2 in, 2 out]
        n34 = Index Array(array=w40, index="Stl File") -> (element=w37:string)
        n35 = case shown="True" w38 {
          tunnel: w39 -> [_ w61]
          tunnel: w37 -> [_ w59]
          tunnel: ["" w56] -> w36
          frame False {
          }
          frame True {
            n36 = Build Path(base path=w61, name or relative path=w59) -> (appended path=w62:path)
            n37 = Build Array(w62) -> (w58:path[])
            n38 = call "Get STL dimensions.vi"("Stl Filenames"=w58) -> ("Limits"=→"stl Limits":sgl[][], "stl Files"=w57:string[])  [unwired: 1 out]
            n39 = Index Array(array=w57) -> (element=w56:string)  [unwired: 1 in]
          }
        }
        n40 = global read "Results_plotter_Global.vi" "Legend"() -> (w51:string[])
        n41 = Array Size(array=w51) -> (size(s)=→"No of Series supplied":i32)
        n42 = local write "stl file String"(w36) -> ()
      }
      frame "Sort out page title" {
        n43 = call "DistillTitle.vi"("Plot Summary in"=w89, "Show Channels with range of Values?"="Show Channels with range of Values?", "Indices to include in Page Title"="Values to include in Page Title", "String in"="") -> ("String out"=w93:string, "AvailableVariables"=w87:string[])  [unwired: 6 in]
        n44 = property on="Values to include in Page Title" class="LstBox (strict)"("Item Names"=w87) -> ()  [unwired: 2 in, 2 out]
        n45 = Concatenate Strings("Page Title Pre Block", w93, "Page Title Post Block") -> (w83:string)
        n46 = call "Fast_string_Replace.vi"("Replace match with:"=" and " ("Individual Characters to Remove"), "Input String"=w83, "matchThis"="&" ("Individual Characters to Remove")) -> ("Output String"=w80:string)  [unwired: 1 in, 1 out]
        n47 = call "Any_Char_Remove.vi"("Individual Characters to Remove"="{}^&", "String in"=w80) -> ("String out"=→"Final Title":string)  [unwired: 1 in]
      }
      frame "Sort plot points" {
        # "Gnuplot   uses 1/1/1970 as its datum time rather than the labview value of 1/1/1904 which is 2082844800 seconds different"
        n48 = call "TimeWizard_NoSearch.vi"("Time/Date Format"="Time/Date Format", "Select Time Zone"="Select Time Zone") -> ("Format String"=→"Time Format String":string, "Formatted date/time string"=→"Formatted date/time string":string, "TZ Shift (hrs)"=→"TZ Shift (hrs)":string, "TZ Shift (sec)"=w96:dbl)  [unwired: 1 in]
        n49 = for {
          tunnel: w105 -> [w116] mode=indexing
          tunnel: [w117] -> w104 mode=indexing
          tunnel: [w109] -> w107 mode=indexing
          tunnel: w96 -> [w108]
          n50 = Unbundle(w116) -> (w112:dbl[], w113:dbl[])
          n51 = Array Max & Min(array=w112) -> (max value=w115:dbl)  [unwired: 3 out]
          n52 = Greater?(x=w115, y=2680560000.0) -> (0:w110:bool)
          n53 = case shown="True" w110 {
            tunnel: w112 -> [w119 w125]
            tunnel: [w119 w121] -> w111
            tunnel: [FALSE TRUE] -> w109
            tunnel: w108 -> [_ w120]
            frame False {
            }
            frame True {
              w124 = 2082844800.0  # datumOffset(s)
              n54 = Subtract(x=w125, y=w124) -> (x-y=w123:dbl[])
              n55 = Add(x=w123, y=w120) -> (x+y=w121:dbl[])
            }
          }
          n56 = Bundle(w111, w113) -> (w117:cluster{dbl[], dbl[]})  [unwired: 1 out]
        }
        n57 = Or Array Elements(Boolean array=w107) -> (logical OR=→"Time format?":bool)
      }
      frame "MakePlotTitles" {
        n58 = call "Create_individual_plot_Titles.vi"("Swop Series and Plots"="Swop Series and Plots") -> ("1D Plot Titles"=w128:string[], "Desired Legends"=w132:string[][], "Plot Legends Auto"=w134:string[], "Dont show axis label"=→"Dont show axis label":bool)  [unwired: 2 in, 1 out]
        n59 = call "Remove_Legend3.vi"("Ordinate Strings"=w134) -> ("Array"=→"Plot Legends Auto":string[])
        n60 = global read "Results_plotter_Global.vi" "Legend"() -> (w133:string[])
        n61 = for {
          tunnel: w132 -> [w143] mode=indexing
          tunnel: w133 -> [w145]
          tunnel: w130 -> [w144]
          tunnel: [w143] -> w131 mode=indexing if=w139
          tunnel: [w142] -> w129 mode=indexing if=w139
          tunnel: w128 -> [w142] mode=indexing
          tunnel: "Only Show Plots with ALL Series" -> [w141]
          n62 = for {
            tunnel: w143 -> [w157] mode=indexing
            tunnel: w145 -> [w156]
            tunnel: w144 -> [w154]
            tunnel: [w150] -> w140 mode=indexing
            n63 = Search 1D Array(1D array=w156, element=w157) -> (index of element=w155:i32)  [unwired: 1 in]
            n64 = Index Array(array=w154, index=w155) -> (element=w153:cluster{dbl[], dbl[]})
            n65 = Unbundle(w153) -> (w152:dbl[])  [unwired: 1 out]
            n66 = Array Size(array=w152) -> (size(s)=w151:i32)
            n67 = Greater Than 0?(x=w151) -> (x > 0?=w150:bool)
          }
          n68 = case shown="True" w141 {
            tunnel: w140 -> [w147 w149]
            tunnel: [w146 w148] -> w139
            frame False {
              n69 = Or Array Elements(Boolean array=w147) -> (logical OR=w146:bool)
            }
            frame True {
              n70 = And Array Elements(Boolean array=w149) -> (logical AND=w148:bool)
            }
          }
        }
        "Desired Legends" <- w131
        "Plot Titles" <- w129
      }
      frame "Save Data files" {
        n71 = local read "Desired Legends"() -> (w160:string[][])
        n72 = Array Size(array=w160) -> (size(s)=w159:i32[])
        n73 = Index Array(array=w159) -> (element=w158:i32)  [unwired: 1 in]
        n74 = for {
          tunnel: w194 -> [w241]
          tunnel: w160 -> [w240] mode=indexing
          tunnel: w179 -> [w239]
          shift-right: [w238] -> _
          shift-left: 1 -> [w237]
          tunnel: [w237] -> w177
          tunnel: [w236] -> w176 mode=indexing
          tunnel: [w234] -> w170 mode=indexing
          tunnel: [w233] -> w169 mode=indexing
          tunnel: [w232] -> w168 mode=indexing
          tunnel: [w231] -> w167 mode=indexing
          tunnel: [w228] -> w166 mode=concatenating
          shift-right: [w227] -> w164
          shift-left: "" -> [w225]
          tunnel: w158 -> [w221]
          i -> [w220]
          n75 = Increment(x=w220) -> (x+1=w222:i32)
          n76 = local read "xAxisBounds"() -> (w229:T7)
          n77 = local read "yAxisBounds"() -> (w230:T7)
          n78 = Equal?(x=w221, y=w222) -> (x = y?=w223:bool)
          n79 = Select(t=-1, s=w223, f=w220) -> (s? t:f=w219:i32)
          n80 = call "MakeDataFileForMultiplot_MATLAB.vi"("Desired Legends"=w240, "1D Folder"=w239, "Plot Array"=w241, "xAxisBounds"=w229, "yAxisBounds"=w230, "Interation number"=w219, "Plot Number"=w237, "Error Bar Type"="Error Bar Type") -> ("Data Directories"=w228:string[], "Plot Array"=w236:i32[], "X Label"=w232:string, "Max Min array"=w234:dbl[][], "Error Bars"=w233:bool[], "File String"=w226:string, "Y Label"=w231:string, "Plot Number 2"=w238:i32)
          n81 = Concatenate Strings(w225, w226) -> (w227:string)
        }
        "Number of Figures" <- w177
        "Plot Array initial" <- w176
        "Max Min array" <- w170
        "Error Bars" <- w169
        "Y Names" <- w167
        "X Names" <- w168
        n82 = Build Array("Column Name", "Numeric Tolerance", "Range of Values") -> (w191:string[])
        n83 = Array Subset(array=w183, length (col)=3 ("length")) -> (w186:string[][])  [unwired: 3 in]
        n84 = Build Array (concatenate)(w191, w186) -> (w184:string[][])
        n85 = for {
          shift-right: [w209] -> w180
          shift-left: "" -> [w206]
          tunnel: w184 -> [w210] mode=indexing
          n86 = for {
            shift-right: [w211] -> w208
            shift-left: w206 -> [w218]
            tunnel: w210 -> [w212] mode=indexing
            i -> [w217]
            n87 = Equal To 0?(x=w217) -> (x = 0?=w216:bool)
            n88 = Select(t="#", s=w216, f="\t") -> (s? t:f=w213:string)
            n89 = Concatenate Strings(w218, w213, w212) -> (w211:string)
          }
          n90 = Concatenate Strings(w208, "\n") -> (w209:string)
        }
        n91 = call "Analyse_string_array.vi"("String array"=w166) -> ("Unique strings"=→"Plot Folder":string[])  [unwired: 1 in, 1 out]
        n92 = feedback-in #1(w164) -> ()
        n93 = feedback #1() -> (w163:string)  [unwired: 1 in]
        n94 = Equal?(x=w164, y=w163) -> (x = y?=→"Duplicate Plot":bool)
        n95 = Build Path(base path=w179, name or relative path="Plot Summary.xls") -> (appended path=w181:path)
        n96 = case shown="True" w175 {
          tunnel: w176 -> [w195 w202]
          tunnel: [w195 w201] -> w172
          frame False {
          }
          frame True {
            n97 = Array Size(array=w202) -> (size(s)=w205:i32[])
            n98 = Index Array(array=w205, index=1) -> (element=w203:i32)
            n99 = Decrement(x=w203) -> (x-1=w200:i32)
            n100 = Initialize Array(-1 ("element"), w200) -> (w198:i32[])
            n101 = Build Array (concatenate)(10000 ("element"), w198) -> (w196:i32[])
            n102 = Build Array (concatenate)(w202, w196) -> (w201:i32[][])
          }
        }
        "Plot Array" <- w172
        n103 = Write to Text File(file (use dialog)=w181, text=w180) -> ()  [unwired: 2 in, 3 out]
        n104 = Array Size(array=w172) -> (size(s)=w174:i32[])
        n105 = Index Array(array=w174, index=1) -> (element=→"No of Series":i32)
      }
      frame "Sort out plot layout" {
        # "Col"
        # "Rows"
        # "Col"
        # "Rows"
        n106 = stacked-sequence {
          seq-local: [_ w297 _ _ _ _ _] -> [_ _ w305 _ _ _ _]
          seq-local: [_ w296 _ _ _ _ _] -> [_ _ w303 _ _ _ _]
          seq-local: [_ _ w306 _ _ _ _] -> [_ _ _ w599 w651 _ _]
          seq-local: [_ _ w304 _ _ _ _] -> [_ _ _ w600 w652 _ w694]
          seq-local: [_ w294 _ _ _ _ _] -> [_ _ w302 _ w654 _ _]
          seq-local: [_ w293 _ _ _ _ _] -> [_ _ _ w596 _ _ _]
          tunnel: w245 -> [_ w295 _ _ _ _ _]
          tunnel: w244 -> [_ _ _ _ _ w680 _]
          tunnel: [_ "Create Input file" _ _ _ _ _] -> w243
          tunnel: w242 -> [_ _ _ w592 _ _ _]
          frame #0 {
            w249 = dbl[] []
            n107 = local read "Max Min array"() -> (w248:dbl[][][])
            n108 = for {
              shift-right: [w267] -> w261
              shift-left: w249 -> [w268]
              shift-right: [w264] -> w251
              shift-left: w249 -> [w266]
              shift-right: [w263] -> w250
              shift-left: w249 -> [w265]
              tunnel: w248 -> [w262] mode=indexing
              n109 = for {
                shift-right: [w275] -> w267
                shift-left: w268 -> [w276]
                shift-right: [w274] -> w264
                shift-left: w266 -> [w273]
                shift-right: [w272] -> w263
                shift-left: w265 -> [w271]
                tunnel: w262 -> [w269] mode=indexing
                i -> [w270]
                n110 = case shown="0, Default" w270 {
                  tunnel: w276 -> [w281 w286 w291]
                  tunnel: w269 -> [w280 w284 w289]
                  tunnel: [w279 w286 w291] -> w275
                  tunnel: [w278 w283 w287] -> w274
                  tunnel: w273 -> [w278 w285 w287]
                  tunnel: [w277 w282 w288] -> w272
                  tunnel: w271 -> [w277 w282 w290]
                  frame 0, Default {
                    n111 = Build Array (concatenate)(w281, w280) -> (w279:dbl[])
                  }
                  frame 1 {
                    n112 = Build Array (concatenate)(w285, w284) -> (w283:dbl[])
                  }
                  frame 2 {
                    n113 = Build Array (concatenate)(w290, w289) -> (w288:dbl[])
                  }
                }
              }
            }
            n114 = Array Max & Min(array=w261) -> (max value=w260:dbl, min value=w258:dbl)  [unwired: 2 out]
            n115 = Array Max & Min(array=w251) -> (max value=w256:dbl, min value=w257:dbl)  [unwired: 2 out]
            n116 = Array Max & Min(array=w250) -> (max value=w255:dbl, min value=w254:dbl)  [unwired: 2 out]
            n117 = Build Array(w260, w258) -> (→"X Pos":dbl[])
            n118 = Build Array(w256, w257) -> (→"Y Pos":dbl[])
            n119 = Build Array(w255, w254) -> (→"Z Pos":dbl[])
          }
          frame #1 {
            n120 = local read "Number of Figures"() -> (w293:i32)
            n121 = local read "nCols"() -> (w296:u8)
            n122 = local read "nRows"() -> (w297:u8)
            n123 = case shown="False" w295 {
              tunnel: w293 -> [w298 w300]
              tunnel: [w298 w299] -> w294
              frame False {
              }
              frame True {
                n124 = Increment(x=w300) -> (x+1=w299:i32)
              }
            }
          }
          frame #2 {
            n125 = case shown="True" "Auto" {
              tunnel: w302 -> [_ w312]
              tunnel: [w308 w311] -> w306
              tunnel: w305 -> [w308 _]
              tunnel: [w307 w310] -> w304
              tunnel: w303 -> [w307 _]
              frame False {
              }
              frame True {
                n126 = case shown="9" w312 {
                  tunnel: [u8 1 ("nRows") w319 w329 w346 w363 w387 w411 w435 w459 w476 w500 w524 w548 w565 w578 u8 5 ("nRows") u8 6 ("nRows")] -> w310
                  tunnel: [u8 1 ("nRows") w318 w328 w345 w362 w386 w410 w434 w458 w475 w499 w523 w547 w564 w577 u8 5 ("nRows") u8 5 ("nRows")] -> w311
                  tunnel: "Horizontal/Vertical plot ratio" -> [_ w317 w325 w342 w359 w383 w407 w431 w455 w472 w496 w520 w544 w561 w579 _ _]
                  frame 1 {
                  }
                  frame 2 {
                    n127 = Greater?(x=w317, y=1.9) -> (0:w315:bool)
                    n128 = case shown="True" w315 {
                      tunnel: [u8 2 ("nRows") u8 1 ("nRows")] -> w319
                      tunnel: [u8 1 ("nRows") u8 2 ("nRows")] -> w318
                      frame False {
                      }
                      frame True {
                      }
                    }
                  }
                  frame 3 {
                    w324 = 3.0 ("upper limit")
                    n129 = In Range and Coerce(upper limit=w324, x=w325, lower limit=1.2) -> (In Range?=w326:bool)  [unwired: 1 out]
                    n130 = case shown="False" w326 {
                      tunnel: [w330 u8 2 ("nRows")] -> w329
                      tunnel: [w331 u8 2 ("nRows")] -> w328
                      tunnel: w325 -> [w334 _]
                      tunnel: w324 -> [w333 _]
                      frame False {
                        n131 = Greater?(x=w334, y=w333) -> (0:w332:bool)
                        n132 = case shown="False" w332 {
                          tunnel: [u8 3 ("nRows") u8 1 ("nRows")] -> w331
                          tunnel: [u8 1 ("nRows") u8 3 ("nRows")] -> w330
                          frame True {
                          }
                          frame False {
                          }
                        }
                      }
                      frame True {
                      }
                    }
                  }
                  frame 4 {
                    w341 = 4.5 ("upper limit")
                    n133 = In Range and Coerce(upper limit=w341, x=w342, lower limit=0.89) -> (In Range?=w343:bool)  [unwired: 1 out]
                    n134 = case shown="False" w343 {
                      tunnel: [w347 u8 2 ("nRows")] -> w346
                      tunnel: [w348 u8 2 ("nRows")] -> w345
                      tunnel: w342 -> [w351 _]
                      tunnel: w341 -> [w350 _]
                      frame False {
                        n135 = Greater?(x=w351, y=w350) -> (0:w349:bool)
                        n136 = case shown="False" w349 {
                          tunnel: [u8 4 ("nRows") u8 1 ("nRows")] -> w348
                          tunnel: [u8 1 ("nRows") u8 4 ("nRows")] -> w347
                          frame True {
                          }
                          frame False {
                          }
                        }
                      }
                      frame True {
                      }
                    }
                  }
                  frame 5 {
                    w358 = 6.7 ("upper limit")
                    n137 = In Range and Coerce(upper limit=w358, x=w359, lower limit=0.73) -> (In Range?=w360:bool)  [unwired: 1 out]
                    n138 = case shown="True" w360 {
                      tunnel: [w364 w377] -> w363
                      tunnel: [w365 w376] -> w362
                      tunnel: w359 -> [w368 w375]
                      tunnel: w358 -> [w367 _]
                      frame False {
                        n139 = Greater?(x=w368, y=w367) -> (0:w366:bool)
                        n140 = case shown="True" w366 {
                          tunnel: [u8 5 ("nRows") u8 1 ("nRows")] -> w365
                          tunnel: [u8 1 ("nRows") u8 5 ("nRows")] -> w364
                          frame True {
                          }
                          frame False {
                          }
                        }
                      }
                      frame True {
                        n141 = Greater?(x=w375, y=2.5) -> (0:w373:bool)
                        n142 = case shown="False" w373 {
                          tunnel: [u8 2 ("nRows") u8 3 ("nRows")] -> w377
                          tunnel: [u8 3 ("nRows") u8 2 ("nRows")] -> w376
                          frame True {
                          }
                          frame False {
                          }
                        }
                      }
                    }
                  }
                  frame 6 {
                    w382 = 8.2 ("upper limit")
                    n143 = In Range and Coerce(upper limit=w382, x=w383, lower limit=0.59) -> (In Range?=w384:bool)  [unwired: 1 out]
                    n144 = case shown="True" w384 {
                      tunnel: [w388 w401] -> w387
                      tunnel: [w389 w400] -> w386
                      tunnel: w383 -> [w392 w399]
                      tunnel: w382 -> [w391 _]
                      frame False {
                        n145 = Greater?(x=w392, y=w391) -> (0:w390:bool)
                        n146 = case shown="False" w390 {
                          tunnel: [u8 6 ("nRows") u8 1 ("nRows")] -> w389
                          tunnel: [u8 1 ("nRows") u8 6 ("nRows")] -> w388
                          frame True {
                          }
                          frame False {
                          }
                        }
                      }
                      frame True {
                        n147 = Greater?(x=w399, y=2.5) -> (0:w397:bool)
                        n148 = case shown="False" w397 {
                          tunnel: [u8 2 ("nRows") u8 3 ("nRows")] -> w401
                          tunnel: [u8 3 ("nRows") u8 2 ("nRows")] -> w400
                          frame True {
                          }
                          frame False {
                          }
                        }
                      }
                    }
                  }
                  frame 7 {
                    w406 = 11.0 ("upper limit")
                    n149 = In Range and Coerce(upper limit=w406, x=w407, lower limit=0.5) -> (In Range?=w408:bool)  [unwired: 1 out]
                    n150 = case shown="True" w408 {
                      tunnel: [w412 w425] -> w411
                      tunnel: [w413 w424] -> w410
                      tunnel: w407 -> [w416 w423]
                      tunnel: w406 -> [w415 _]
                      frame False {
                        n151 = Greater?(x=w416, y=w415) -> (0:w414:bool)
                        n152 = case shown="True" w414 {
                          tunnel: [u8 7 ("nRows") u8 1 ("nRows")] -> w413
                          tunnel: [u8 1 ("nRows") u8 7 ("nRows")] -> w412
                          frame True {
                          }
                          frame False {
                          }
                        }
                      }
                      frame True {
                        n153 = Greater?(x=w423, y=2.5) -> (0:w421:bool)
                        n154 = case shown="True" w421 {
                          tunnel: [u8 2 ("nRows") u8 4 ("nRows")] -> w425
                          tunnel: [u8 4 ("nRows") u8 2 ("nRows")] -> w424
                          frame True {
                          }
                          frame False {
                          }
                        }
                      }
                    }
                  }
                  frame 8 {
                    w430 = 14.0 ("upper limit")
                    n155 = In Range and Coerce(upper limit=w430, x=w431, lower limit=0.45) -> (In Range?=w432:bool)  [unwired: 1 out]
                    n156 = case shown="True" w432 {
                      tunnel: [w436 w449] -> w435
                      tunnel: [w437 w448] -> w434
                      tunnel: w431 -> [w440 w447]
                      tunnel: w430 -> [w439 _]
                      frame False {
                        n157 = Greater?(x=w440, y=w439) -> (0:w438:bool)
                        n158 = case shown="False" w438 {
                          tunnel: [u8 8 ("nRows") u8 1 ("nRows")] -> w437
                          tunnel: [u8 1 ("nRows") u8 8 ("nRows")] -> w436
                          frame True {
                          }
                          frame False {
                          }
                        }
                      }
                      frame True {
                        n159 = Greater?(x=w447, y=2.1) -> (0:w445:bool)
                        n160 = case shown="True" w445 {
                          tunnel: [u8 2 ("nRows") u8 4 ("nRows")] -> w449
                          tunnel: [u8 4 ("nRows") u8 2 ("nRows")] -> w448
                          frame True {
                          }
                          frame False {
                          }
                        }
                      }
                    }
                  }
                  frame 9 {
                    w454 = 1.5 ("upper limit")
                    n161 = In Range and Coerce(upper limit=w454, x=w455, lower limit=0.7) -> (In Range?=w456:bool)  [unwired: 1 out]
                    n162 = case shown="False" w456 {
                      tunnel: [w460 u8 3 ("nRows")] -> w459
                      tunnel: [w461 u8 3 ("nRows")] -> w458
                      tunnel: w455 -> [w464 _]
                      tunnel: w454 -> [w463 _]
                      frame False {
                        n163 = Greater?(x=w464, y=w463) -> (0:w462:bool)
                        n164 = case shown="True" w462 {
                          tunnel: [u8 5 ("nRows") u8 2 ("nRows")] -> w461
                          tunnel: [u8 2 ("nRows") u8 5 ("nRows")] -> w460
                          frame True {
                          }
                          frame False {
                          }
                        }
                      }
                      frame True {
                      }
                    }
                  }
                  frame 10 {
                    w471 = 3.9 ("upper limit")
                    n165 = In Range and Coerce(upper limit=w471, x=w472, lower limit=1.12) -> (In Range?=w473:bool)  [unwired: 1 out]
                    n166 = case shown="False" w473 {
                      tunnel: [w477 w490] -> w476
                      tunnel: [w478 w489] -> w475
                      tunnel: w472 -> [w481 w488]
                      tunnel: w471 -> [w480 _]
                      frame False {
                        n167 = Greater?(x=w481, y=w480) -> (0:w479:bool)
                        n168 = case shown="False" w479 {
                          tunnel: [u8 5 ("nRows") u8 2 ("nRows")] -> w478
                          tunnel: [u8 2 ("nRows") u8 5 ("nRows")] -> w477
                          frame True {
                          }
                          frame False {
                          }
                        }
                      }
                      frame True {
                        n169 = Greater?(x=w488, y=2.1) -> (0:w486:bool)
                        n170 = case shown="False" w486 {
                          tunnel: [u8 3 ("nRows") u8 4 ("nRows")] -> w490
                          tunnel: [u8 4 ("nRows") u8 3 ("nRows")] -> w489
                          frame True {
                          }
                          frame False {
                          }
                        }
                      }
                    }
                  }
                  frame 11 {
                    w495 = 4.1 ("upper limit")
                    n171 = In Range and Coerce(upper limit=w495, x=w496, lower limit=0.94) -> (In Range?=w497:bool)  [unwired: 1 out]
                    n172 = case shown="True" w497 {
                      tunnel: [w501 w514] -> w500
                      tunnel: [w502 w513] -> w499
                      tunnel: w496 -> [w505 w512]
                      tunnel: w495 -> [w504 _]
                      frame False {
                        n173 = Greater?(x=w505, y=w504) -> (0:w503:bool)
                        n174 = case shown="True" w503 {
                          tunnel: [u8 6 ("nRows") u8 2 ("nRows")] -> w502
                          tunnel: [u8 2 ("nRows") u8 6 ("nRows")] -> w501
                          frame True {
                          }
                          frame False {
                          }
                        }
                      }
                      frame True {
                        n175 = Greater?(x=w512, y=2.1) -> (0:w510:bool)
                        n176 = case shown="False" w510 {
                          tunnel: [u8 3 ("nRows") u8 4 ("nRows")] -> w514
                          tunnel: [u8 4 ("nRows") u8 3 ("nRows")] -> w513
                          frame True {
                          }
                          frame False {
                          }
                        }
                      }
                    }
                  }
                  frame 12 {
                    w519 = 5.6 ("upper limit")
                    n177 = In Range and Coerce(upper limit=w519, x=w520, lower limit=0.94) -> (In Range?=w521:bool)  [unwired: 1 out]
                    n178 = case shown="False" w521 {
                      tunnel: [w525 w538] -> w524
                      tunnel: [w526 w537] -> w523
                      tunnel: w520 -> [w529 w536]
                      tunnel: w519 -> [w528 _]
                      frame False {
                        n179 = Greater?(x=w529, y=w528) -> (0:w527:bool)
                        n180 = case shown="False" w527 {
                          tunnel: [u8 6 ("nRows") u8 2 ("nRows")] -> w526
                          tunnel: [u8 2 ("nRows") u8 6 ("nRows")] -> w525
                          frame True {
                          }
                          frame False {
                          }
                        }
                      }
                      frame True {
                        n181 = Greater?(x=w536, y=2.1) -> (0:w534:bool)
                        n182 = case shown="False" w534 {
                          tunnel: [u8 3 ("nRows") u8 4 ("nRows")] -> w538
                          tunnel: [u8 4 ("nRows") u8 3 ("nRows")] -> w537
                          frame True {
                          }
                          frame False {
                          }
                        }
                      }
                    }
                  }
                  frame 13, 14 {
                    w543 = 5.3 ("upper limit")
                    n183 = In Range and Coerce(upper limit=w543, x=w544, lower limit=1.15) -> (In Range?=w545:bool)  [unwired: 1 out]
                    n184 = case shown="False" w545 {
                      tunnel: [w549 u8 4 ("nRows")] -> w548
                      tunnel: [w550 u8 4 ("nRows")] -> w547
                      tunnel: w544 -> [w553 _]
                      tunnel: w543 -> [w552 _]
                      frame False {
                        n185 = Greater?(x=w553, y=w552) -> (0:w551:bool)
                        n186 = case shown="True" w551 {
                          tunnel: [u8 7 ("nRows") u8 2 ("nRows")] -> w550
                          tunnel: [u8 2 ("nRows") u8 7 ("nRows")] -> w549
                          frame True {
                          }
                          frame False {
                          }
                        }
                      }
                      frame True {
                      }
                    }
                  }
                  frame 15, 16 {
                    w560 = 7.5 ("upper limit")
                    n187 = In Range and Coerce(upper limit=w560, x=w561, lower limit=0.98) -> (In Range?=w562:bool)  [unwired: 1 out]
                    n188 = case shown="True" w562 {
                      tunnel: [w566 u8 4 ("nRows")] -> w565
                      tunnel: [w567 u8 4 ("nRows")] -> w564
                      tunnel: w561 -> [w570 _]
                      tunnel: w560 -> [w569 _]
                      frame False {
                        n189 = Greater?(x=w570, y=w569) -> (0:w568:bool)
                        n190 = case shown="False" w568 {
                          tunnel: [u8 8 ("nRows") u8 2 ("nRows")] -> w567
                          tunnel: [u8 2 ("nRows") u8 8 ("nRows")] -> w566
                          frame True {
                          }
                          frame False {
                          }
                        }
                      }
                      frame True {
                      }
                    }
                  }
                  frame 17..20 {
                    n191 = Greater?(x=w579, y=1.9) -> (0:w580:bool)
                    n192 = case shown="True" w580 {
                      tunnel: [u8 5 ("nRows") u8 4 ("nRows")] -> w578
                      tunnel: [u8 4 ("nRows") u8 5 ("nRows")] -> w577
                      frame False {
                      }
                      frame True {
                      }
                    }
                  }
                  frame 21..25 {
                  }
                  frame 26, Default {
                  }
                }
              }
            }
          }
          frame #3 {
            n193 = local write "nRows"(w599) -> ()
            n194 = local write "nCols"(w600) -> ()
            n195 = for {
              N: w599 -> [_]
              tunnel: w600 -> [w641]
              tunnel: w596 -> [w640]
              tunnel: [w639] -> w601 mode=indexing
              tunnel: [w637] -> w595 mode=concatenating
              i -> [w642]
              n196 = Multiply(x=w641, y=w642) -> (x*y=w638:i32)
              n197 = for {
                N: w641 -> [_]
                tunnel: w638 -> [w650]
                tunnel: w640 -> [w649]
                tunnel: [w643] -> w639 mode=indexing
                tunnel: [w647] -> w637 mode=indexing
                i -> [w648]
                n198 = Add(x=w650, y=w648) -> (x+y=w645:i32)
                n199 = Equal To 0?(x=w648) -> (x = 0?=w647:bool)
                n200 = Less?(x=w645, y=w649) -> (x < y?=w646:bool)
                n201 = Select(t=w645, s=w646, f=-1) -> (s? t:f=w643:i32)
              }
            }
            n202 = Decrement(x=w599) -> (x-1=w598:u8)
            n203 = local read "Dont show axis label"() -> (w593:bool)
            n204 = for {
              N: w600 -> [_]
              tunnel: w601 -> [w627]
              tunnel: w598 -> [w629]
              tunnel: [w626] -> w597 mode=indexing
              i -> [w630]
              n205 = Index Array(array=w627, index (row)=w629, index (col)=w630) -> (element=w625:i32)
              n206 = Decrement(x=w629) -> (x-1=w628:u8)
              n207 = Less Than 0?(x=w625) -> (x < 0?=w631:bool)
              n208 = case shown="False" w631 {
                tunnel: w630 -> [_ w636]
                tunnel: w628 -> [_ w635]
                tunnel: w627 -> [_ w634]
                tunnel: [w632 w633] -> w626
                tunnel: w625 -> [w632 _]
                frame False {
                }
                frame True {
                  n209 = Index Array(array=w634, index (row)=w635, index (col)=w636) -> (element=w633:i32)
                }
              }
            }
            n210 = for {
              N: w596 -> [_]
              tunnel: w597 -> [w624]
              tunnel: [w621] -> w590 mode=indexing
              i -> [w623]
              n211 = Search 1D Array(1D array=w624, element=w623) -> (index of element=w622:i32)  [unwired: 1 in]
              n212 = Greater Or Equal To 0?(x=w622) -> (x >= 0?=w621:bool)
            }
            n213 = case shown="False" w593 {
              tunnel: w595 -> [w603 w608]
              tunnel: [w603 w607] -> w594
              tunnel: w592 -> [_ w606]
              tunnel: [w602 w605] -> w591
              tunnel: w590 -> [w602 w604]
              frame False {
              }
              frame True {
                n214 = case shown="True" w606 {
                  tunnel: w608 -> [w611 w615]
                  tunnel: [w610 w615] -> w607
                  tunnel: [w609 w616] -> w605
                  tunnel: w604 -> [w609 w617]
                  frame False {
                    n215 = for {
                      tunnel: w611 -> [w613] mode=indexing
                      tunnel: [w612] -> w610 mode=indexing
                      n216 = And(x=w613, y=FALSE) -> (x .and. y?=w612:bool)
                    }
                  }
                  frame True {
                    n217 = for {
                      tunnel: w617 -> [w619] mode=indexing
                      tunnel: [w618] -> w616 mode=indexing
                      n218 = And(x=w619, y=FALSE) -> (x .and. y?=w618:bool)
                    }
                  }
                }
              }
            }
            "Y labels" <- w594
            "X Labels" <- w591
          }
          frame #4 {
            n219 = Multiply(x=w651, y=w652) -> (x*y=w656:u8)
            n220 = Equal?(x=w654, y=w656) -> (x = y?=w655:bool)
            n221 = case shown="False" w655 {
              tunnel: [w666 "0.5;0.04" ("Main Title")] -> w653
              tunnel: w652 -> [w675 _]
              tunnel: w651 -> [w665 _]
              frame False {
                w674 = 1.0 ("x")
                n222 = Divide(x=1.0, y=w665) -> (x/y=w663:dbl)
                n223 = Divide(x=w674, y=w675) -> (x/y=w658:dbl)
                n224 = Multiply(x=w663, y=0.3) -> (x*y=w662:dbl)
                n225 = Multiply(x=w658, y=0.3) -> (x*y=w659:dbl)
                n226 = Subtract(x=w663, y=w662) -> (x-y=w661:dbl)
                n227 = Subtract(x=w658, y=w659) -> (x-y=w657:dbl)
                n228 = Subtract(x=w674, y=w657) -> (x-y=w673:dbl)
                n229 = Number To Fractional String(number=w673, precision (6)=i16 2) -> (F-format string=w670:string)  [unwired: 2 in]
                n230 = Number To Fractional String(number=w661, precision (6)=i16 2) -> (F-format string=w667:string)  [unwired: 2 in]
                n231 = Concatenate Strings(w670, ";" ("Main Title"), w667) -> (w666:string)
              }
              frame True {
              }
            }
            "Legend Location" <- w653
          }
          frame #5 {
            n232 = global read "Results_plotter_Global.vi" "3D Ch Names"() -> (w679:string[])
            n233 = Index Array(array=w679, index=3) -> (element=w677:string)
            n234 = Index Array(array=w680, index (col)=2 ("disabled index (col)")) -> (element=w684:string[])  [unwired: 1 in]
            n235 = Index Array(array=w680, index (col)=0 ("disabled index (col)")) -> (element=w685:string[])  [unwired: 1 in]
            n236 = Search 1D Array(1D array=w685, element=w677) -> (index of element=w686:i32)  [unwired: 1 in]
            n237 = Index Array(array=w684, index=w686) -> (element=w688:string)
            n238 = Fract/Exp String To Number(string=w688, default (0 dbl)=nan ("default (0 DBL)")) -> (number=w690:dbl)  [unwired: 2 in, 1 out]
            n239 = Negate(x=w690) -> (-x=w691:dbl)
            n240 = Format Into String(format string="0;0;%.3f", w691) -> (resulting string=→"ILocationRotations":string)  [unwired: 2 in, 1 out]
          }
          frame #6 {
            n241 = local read "Plot Titles"() -> (w697:string[])
            n242 = Divide(x=100, y=w694) -> (x/y=w693:dbl)
            n243 = call "Reduce Title length.vi"("Reduce Individual Plot Title Lengths if too long"="Reduce Individual Plot Title Lengths if too long", "Array in"=w697, "No of Charcters"=w693) -> ("Array out"=w696:string[])  [unwired: 2 in]
            n244 = local write "Plot Titles"(w696) -> ()
          }
        }
      }
      frame "Create Input file" {
        n245 = local read "Error Bars"() -> (w698:bool[][])
        n246 = local read "Plotstyles"() -> (w704:T2[])
        n247 = local read "Plot Array"() -> (w712:i32[][])
        n248 = Index Array(array=w708, index (col)=1 ("disabled index (col)")) -> (element=w706:string[])  [unwired: 1 in]
        n249 = Index Array(array=w708, index (col)=0 ("disabled index (col)")) -> (element=w707:string[])  [unwired: 1 in]
        n250 = for {
          tunnel: w712 -> [w727] mode=indexing
          shift-right: [w726] -> _
          shift-left: 0 -> [w717]
          tunnel: w707 -> [w724]
          tunnel: [w718] -> w705 mode=concatenating if=w722
          tunnel: w706 -> [w723]
          tunnel: w704 -> [w720]
          tunnel: w703 -> [w719]
          tunnel: w700 -> [w715]
          tunnel: w699 -> [w714]
          tunnel: w698 -> [w713] mode=indexing
          i -> [w721]
          n251 = Increment(x=w717) -> (x+1=w716:i32)
          n252 = for {
            shift-right: [w744] -> w725
            shift-left: 0 -> [w732]
            tunnel: w727 -> [w737] mode=indexing
            tunnel: w724 -> [w743]
            tunnel: [w742] -> w718 mode=indexing if=w740
            tunnel: w723 -> [w741]
            tunnel: w716 -> [w739]
            tunnel: w721 -> [w738]
            tunnel: w720 -> [w735]
            tunnel: w719 -> [w734]
            tunnel: w715 -> [w731]
            tunnel: w714 -> [w730]
            tunnel: w713 -> [w729] mode=indexing
            i -> [w736]
            n253 = Greater Or Equal To 0?(x=w737) -> (x >= 0?=w740:bool)
            n254 = Increment(x=w732) -> (x+1=w733:i32)
            n255 = for {
              tunnel: w743 -> [w757] mode=indexing
              tunnel: [w756] -> w742 mode=indexing
              tunnel: w741 -> [w755] mode=indexing
              tunnel: w733 -> [w754]
              tunnel: w739 -> [w753]
              tunnel: w738 -> [w752]
              tunnel: w737 -> [w751]
              tunnel: w736 -> [w750]
              tunnel: w735 -> [w749]
              tunnel: w734 -> [w748]
              tunnel: w731 -> [w747]
              tunnel: w730 -> [w746]
              tunnel: w729 -> [w745]
              n256 = case shown="\"lLocationRotations\"" w757 {
                tunnel: [w759 w771 w792 w804 w810 w840 w870 w906 w910 w916 w935 w940 w958 w965 w975 "stl file String" w986 "lRefArrowBaseCoord" "lRefArrowColor" "lRefArrowComponents" "lRefArrowSize" "lRefPointColor" "lRefPointCoord" "lRefPointSize" "View Angle" "Font Size" w1008 w1009 w1019 w1021 "Legend Title" w1023 "MainTitleFontSize" w1026 w1033 w1036 w1066 w1078 w1093 w1100 w1112 w1123 w1178 w1184 w1187 w1192 w1198 w1202 w1204 w1208] -> w756
                tunnel: w755 -> [_ _ _ _ _ _ _ _ _ _ _ _ _ _ _ _ _ _ _ _ _ _ _ _ _ _ _ _ _ _ _ _ _ _ _ _ _ _ _ _ _ _ _ _ _ _ _ _ _ w1208]
                tunnel: w754 -> [_ _ _ _ _ _ _ _ _ _ _ _ _ _ _ _ _ _ _ _ _ _ _ _ _ _ _ _ _ _ _ _ _ _ _ _ _ _ _ _ _ _ _ _ _ _ _ _ _ _]
                tunnel: w753 -> [_ _ _ _ _ _ _ _ _ _ _ _ _ _ _ _ _ _ _ _ _ _ _ _ _ _ _ _ _ _ _ _ _ _ w1032 _ _ _ _ _ _ _ _ _ _ _ _ _ _ _]
                tunnel: w752 -> [w760 w772 w793 w805 _ _ _ _ _ _ _ _ w959 _ _ _ _ _ _ _ _ _ _ _ _ _ _ _ _ _ _ _ _ _ _ _ _ _ _ _ _ _ _ _ _ _ _ _ _ _]
                tunnel: w751 -> [w758 w770 w791 w803 w809 w839 w869 _ _ w917 w936 w939 _ _ w974 _ _ _ _ _ _ _ _ _ _ _ _ _ _ _ _ _ _ _ _ _ _ w1079 w1094 w1101 _ w1124 _ _ _ _ _ w1203 _ _]
                tunnel: w750 -> [_ _ _ _ _ _ _ _ _ _ _ _ _ _ _ _ _ _ _ _ _ _ _ _ _ _ _ _ _ _ _ _ _ w1031 _ _ _ _ _ _ w1116 _ w1177 w1186 w1190 w1195 w1201 _ w1207 _]
                tunnel: w749 -> [_ _ _ _ _ _ _ _ _ _ _ _ _ _ _ _ _ _ _ _ _ _ _ _ _ _ _ _ _ _ _ _ _ w1025 _ _ _ _ _ _ w1114 _ _ w1183 w1188 w1191 w1199 _ w1205 _]
                tunnel: w748 -> [_ _ _ _ _ _ _ _ _ _ _ _ _ _ _ _ w987 _ _ _ _ _ _ _ _ _ _ _ _ _ _ _ _ _ _ _ _ _ _ _ _ _ _ _ _ _ _ _ _ _]
                tunnel: w747 -> [_ _ _ _ _ _ _ _ _ _ _ _ _ _ _ _ _ _ _ _ _ _ _ _ _ _ _ _ _ _ _ _ _ _ _ _ _ w1080 w1095 _ _ w1125 _ _ _ _ _ _ _ _]
                tunnel: w746 -> [_ _ _ _ _ _ _ _ _ _ _ _ _ _ w973 _ _ _ _ _ _ _ _ _ _ _ _ _ _ _ _ _ _ _ _ _ _ _ _ _ _ _ _ _ _ _ _ _ _ _]
                tunnel: w745 -> [_ _ _ _ _ _ _ w905 w909 _ _ _ _ _ _ _ _ _ _ _ _ _ _ _ _ _ _ _ _ _ _ _ _ _ _ _ _ _ _ _ _ _ _ _ _ _ _ _ _ _]
                frame "fAxisLabelX" {
                  n257 = case shown="10000" w758 {
                    tunnel: w760 -> [w761 _]
                    tunnel: [w764 w768] -> w759
                    frame Default {
                      n258 = local read "X Labels"() -> (w767:bool[])
                      n259 = Index Array(array=w767, index=w761) -> (element=w766:bool)
                      n260 = local read "X Names"() -> (w763:string[])
                      n261 = Index Array(array=w763, index=w761) -> (element=w762:string)
                      n262 = Select(t=w762, s=w766, f="") -> (s? t:f=w764:string)
                    }
                    frame 10000 {
                      n263 = global read "Results_plotter_Global.vi" "3D Ch Names"() -> (w769:string[])
                      n264 = Index Array(array=w769) -> (element #1=w768:string)  [unwired: 3 in, 2 out]
                    }
                  }
                }
                frame "fTickLabel" {
                  n265 = case shown="Default" w770 {
                    tunnel: w772 -> [w774 _]
                    tunnel: [w775 "1;1;1" ("X Label")] -> w771
                    frame Default {
                      n266 = local read "Set bounds using XY Plot \non Results file plotter"() -> (w773:bool)
                      n267 = case shown="False" w773 {
                        tunnel: ["1;1;1" ("X Label") w784] -> w775
                        tunnel: w774 -> [_ w782]
                        frame False {
                        }
                        frame True {
                          n268 = local read "X Labels"() -> (w789:bool[])
                          n269 = local read "Y labels"() -> (w783:bool[])
                          n270 = Index Array(array=w783, index=w782) -> (element=w779:bool)
                          n271 = Index Array(array=w789, index=w782) -> (element=w788:bool)
                          n272 = Select(t="1", s=w779, f="0") -> (s? t:f=w778:string)
                          n273 = Select(t="1", s=w788, f="0") -> (s? t:f=w785:string)
                          n274 = Format Into String(format string="%s;%s;", w785, w778) -> (resulting string=w784:string)  [unwired: 2 in, 1 out]
                        }
                      }
                    }
                    frame 10000 {
                    }
                  }
                }
                frame "fAxisLabelY" {
                  n275 = case shown="10000" w791 {
                    tunnel: w793 -> [w795 _]
                    tunnel: [w797 w801] -> w792
                    frame Default {
                      n276 = local read "Y labels"() -> (w800:bool[])
                      n277 = Index Array(array=w800, index=w795) -> (element=w799:bool)
                      n278 = local read "Y Names"() -> (w796:string[])
                      n279 = Index Array(array=w796, index=w795) -> (element=w794:string)
                      n280 = Select(t=w794, s=w799, f="") -> (s? t:f=w797:string)
                    }
                    frame 10000 {
                      n281 = global read "Results_plotter_Global.vi" "3D Ch Names"() -> (w802:string[])
                      n282 = Index Array(array=w802) -> (element #2=w801:string)  [unwired: 3 in, 2 out]
                    }
                  }
                }
                frame "fAxisLabelYrightZloc" {
                  n283 = case shown="10000" w803 {
                    tunnel: w805 -> [_ _]
                    tunnel: ["fAxisLabelYright" w807] -> w804
                    frame Default {
                    }
                    frame 10000 {
                      n284 = global read "Results_plotter_Global.vi" "3D Ch Names"() -> (w808:string[])
                      n285 = Index Array(array=w808) -> (element #3=w807:string)  [unwired: 3 in, 2 out]
                    }
                  }
                }
                frame "fAxisLimX" {
                  n286 = case shown="10000" w809 {
                    tunnel: [w811 w829] -> w810
                    frame Default {
                      n287 = local read "xAxisBounds"() -> (w821:T7)
                      n288 = Unbundle By Name(w821) -> ("Min"=w820:T8, "Max"=w819:T8)
                      n289 = Unbundle By Name(w820) -> ("Auto"=w818:bool, "Value"=w817:dbl)
                      n290 = Unbundle By Name(w819) -> ("Auto"=w815:bool, "Value"=w814:dbl)
                      n291 = case shown="True" w818 {
                        tunnel: w817 -> [w826 _]
                        tunnel: [w825 "-inf"] -> w816
                        frame False {
                          n292 = Number To Fractional String(number=w826) -> (F-format string=w825:string)  [unwired: 3 in]
                        }
                        frame True {
                        }
                      }
                      n293 = case shown="True" w815 {
                        tunnel: w814 -> [w823 _]
                        tunnel: [w822 "inf"] -> w813
                        frame False {
                          n294 = Number To Fractional String(number=w823) -> (F-format string=w822:string)  [unwired: 3 in]
                        }
                        frame True {
                        }
                      }
                      n295 = Concatenate Strings(w816, ";" ("string"), w813) -> (w811:string)
                    }
                    frame 10000 {
                      n296 = case shown="True" "X Limits Auto" {
                        tunnel: ["Location X limits" w831] -> w829
                        frame False {
                        }
                        frame True {
                          n297 = local read "stl Limits"() -> (w838:sgl[][])
                          n298 = local read "X Pos"() -> (w836:dbl[])
                          n299 = Index Array(array=w838, index (row)=0) -> (element=w835:sgl[])  [unwired: 1 in]
                          n300 = Build Array (concatenate)(w836, w835) -> (w834:dbl[])
                          n301 = Array Max & Min(array=w834) -> (max value=w833:dbl, min value=w832:dbl)  [unwired: 2 out]
                          n302 = call "Set Plot limits.vi"("Min"=w832, "Max"=w833) -> ("resulting string"=w831:string)
                        }
                      }
                    }
                  }
                }
                frame "fAxisLimY" {
                  n303 = case shown="10000" w839 {
                    tunnel: [w841 w858] -> w840
                    frame Default {
                      n304 = local read "yAxisBounds"() -> (w851:T7)
                      n305 = Unbundle By Name(w851) -> ("Min"=w850:T8, "Max"=w849:T8)
                      n306 = Unbundle By Name(w850) -> ("Auto"=w848:bool, "Value"=w847:dbl)
                      n307 = Unbundle By Name(w849) -> ("Auto"=w845:bool, "Value"=w844:dbl)
                      n308 = case shown="False" w848 {
                        tunnel: w847 -> [w856 _]
                        tunnel: [w855 "-inf"] -> w846
                        frame False {
                          n309 = Number To Fractional String(number=w856) -> (F-format string=w855:string)  [unwired: 3 in]
                        }
                        frame True {
                        }
                      }
                      n310 = case shown="True" w845 {
                        tunnel: w844 -> [w853 _]
                        tunnel: [w852 "inf"] -> w843
                        frame False {
                          n311 = Number To Fractional String(number=w853) -> (F-format string=w852:string)  [unwired: 3 in]
                        }
                        frame True {
                        }
                      }
                      n312 = Concatenate Strings(w846, ";" ("string"), w843) -> (w841:string)
                    }
                    frame 10000 {
                      n313 = case shown="True" "Y Limits Auto" {
                        tunnel: ["Location Y limits" w861] -> w858
                        frame False {
                        }
                        frame True {
                          n314 = local read "stl Limits"() -> (w868:sgl[][])
                          n315 = local read "Y Pos"() -> (w866:dbl[])
                          n316 = Index Array(array=w868, index (row)=1) -> (element=w865:sgl[])  [unwired: 1 in]
                          n317 = Build Array (concatenate)(w866, w865) -> (w864:dbl[])
                          n318 = Array Max & Min(array=w864) -> (max value=w863:dbl, min value=w862:dbl)  [unwired: 2 out]
                          n319 = call "Set Plot limits.vi"("Min"=w862, "Max"=w863) -> ("resulting string"=w861:string)
                        }
                      }
                    }
                  }
                }
                frame "fAxisLimYrightZloc" {
                  n320 = case shown="10000" w869 {
                    tunnel: [w871 w889] -> w870
                    frame Default {
                      n321 = local read "yAxisBounds"() -> (w881:T7)
                      n322 = Unbundle By Name(w881) -> ("Min"=w880:T8, "Max"=w879:T8)
                      n323 = Unbundle By Name(w880) -> ("Auto"=w878:bool, "Value"=w877:dbl)
                      n324 = Unbundle By Name(w879) -> ("Auto"=w875:bool, "Value"=w874:dbl)
                      n325 = case shown="False" w878 {
                        tunnel: w877 -> [w886 _]
                        tunnel: [w885 "-inf"] -> w876
                        frame False {
                          n326 = Number To Fractional String(number=w886) -> (F-format string=w885:string)  [unwired: 3 in]
                        }
                        frame True {
                        }
                      }
                      n327 = case shown="True" w875 {
                        tunnel: w874 -> [w883 _]
                        tunnel: [w882 "inf"] -> w873
                        frame False {
                          n328 = Number To Fractional String(number=w883) -> (F-format string=w882:string)  [unwired: 3 in]
                        }
                        frame True {
                        }
                      }
                      n329 = Concatenate Strings(w876, ";" ("string"), w873) -> (w871:string)
                    }
                    frame 10000 {
                      n330 = case shown="False" "Z Limits Auto" {
                        tunnel: ["Location Z limits" w891] -> w889
                        frame False {
                        }
                        frame True {
                          n331 = local read "stl Limits"() -> (w904:sgl[][])
                          n332 = local read "Z Pos"() -> (w902:dbl[])
                          n333 = Index Array(array=w904, index (row)=2) -> (element=w901:sgl[])  [unwired: 1 in]
                          n334 = Build Array (concatenate)(w902, w901) -> (w900:dbl[])
                          n335 = Array Max & Min(array=w900) -> (max value=w893:dbl, min value=w892:dbl)  [unwired: 2 out]
                          n336 = Subtract(x=w893, y=w892) -> (x-y=w894:dbl)
                          n337 = Divide(x=w894, y=40.0) -> (x/y=w896:dbl)
                          n338 = Subtract(x=w892, y=w896) -> (x-y=w899:dbl)
                          n339 = Add(x=w893, y=w896) -> (x+y=w898:dbl)
                          n340 = Format Into String(format string="%.3e;%.3e", w899, w898) -> (resulting string=w891:string)  [unwired: 2 in, 1 out]
                        }
                      }
                    }
                  }
                }
                frame "fErrorbarColumn" {
                  n341 = Select(t="2" ("Main Title"), s=w905, f="") -> (s? t:f=w906:string)
                }
                frame "fErrorbarOrientation" {
                  n342 = case shown="True" w909 {
                    tunnel: ["none" ("Main Title") w912] -> w910
                    frame False {
                    }
                    frame True {
                      n343 = global read "Results_plotter_Global.vi" "Transpose"() -> (w913:bool)
                      n344 = Select(t="horizontal" ("Main Title"), s=w913, f="vertical" ("Main Title")) -> (s? t:f=w912:string)
                    }
                  }
                }
                frame "fGrid" {
                  n345 = case shown="Default" w917 {
                    tunnel: [w919 "1;1;0" ("Main Title")] -> w916
                    frame Default {
                      n346 = local read "Y/R tics And Grids"() -> (w922:T4)
                      n347 = local read "X/Theta tics And Grids"() -> (w933:T4)
                      n348 = Unbundle By Name(w922) -> ("Grids.Gridlines"=w924:T10)
                      n349 = Unbundle By Name(w933) -> ("Grids.Gridlines"=w931:T10)
                      n350 = Equal?(x=w924, y=T10."No grids" ("Grids.Gridlines")) -> (x = y?=w925:bool)
                      n351 = Equal?(x=w931, y=T10."No grids" ("Grids.Gridlines")) -> (x = y?=w930:bool)
                      n352 = Select(t="0" ("Main Title"), s=w925, f="1" ("Main Title")) -> (s? t:f=w921:string)
                      n353 = Select(t="0" ("Main Title"), s=w930, f="1" ("Main Title")) -> (s? t:f=w920:string)
                      n354 = Concatenate Strings(w920, ";" ("Main Title"), w921) -> (w919:string)
                    }
                    frame 10000 {
                    }
                  }
                }
                frame "fGridMinor" {
                  n355 = case shown="Default" w936 {
                    tunnel: ["0;0" ("Main Title") "0;0;0" ("Main Title")] -> w935
                    frame Default {
                    }
                    frame 10000 {
                    }
                  }
                }
                frame "fLogAxis" {
                  n356 = case shown="Default" w939 {
                    tunnel: [w941 "0;0;0" ("t")] -> w940
                    frame Default {
                      w942 = ";"
                      n357 = Unbundle By Name("Y/R tics And Grids") -> ("Mapping"=w949:enum8{"Lin", "Log"})
                      n358 = Unbundle By Name("X/Theta tics And Grids") -> ("Mapping"=w947:enum8{"Lin", "Log"})
                      n359 = case shown="\"Lin\"" w949 {
                        tunnel: ["0" "1"] -> w948
                        frame "Lin" {
                        }
                        frame "Log" {
                        }
                      }
                      n360 = case shown="\"Lin\"" w947 {
                        tunnel: ["0" "1"] -> w946
                        frame "Lin" {
                        }
                        frame "Log" {
                        }
                      }
                      n361 = case shown="\"Lin\"" "2nd Y Axis" {
                        tunnel: ["0" "1"] -> w943
                        frame "Lin" {
                        }
                        frame "Log" {
                        }
                      }
                      n362 = Concatenate Strings(w946, w942, w948, w942, w943) -> (w941:string)
                    }
                    frame 10000 {
                    }
                  }
                }
                frame "fTitle" {
                  n363 = local read "Plot Titles"() -> (w963:string[])
                  n364 = Select(t=w963, s="Individual Plot Titles", f="ManualPlotTitles") -> (s? t:f=w960:string[])
                  n365 = Index Array(array=w960, index=w959) -> (element=w958:string)
                }
                frame "lListFiguresShown" {
                  n366 = local read "Number of Figures"() -> (w964:i32)
                  n367 = for {
                    N: w964 -> [_]
                    shift-right: [w967] -> w965
                    shift-left: "" -> [w970]
                    i -> [w972]
                    n368 = Increment(x=w972) -> (x+1=w971:i32)
                    n369 = Number To Decimal String(number=w971) -> (decimal integer string=w969:string)  [unwired: 1 in]
                    n370 = Concatenate Strings(w970, w969, ";" ("string")) -> (w967:string)
                  }
                }
                frame "lLocationAct" {
                  n371 = case shown="10000" w974 {
                    tunnel: ["0" w979] -> w975
                    tunnel: w973 -> [_ _]
                    frame Default {
                    }
                    frame 10000 {
                      n372 = local read "stl file String"() -> (w978:string)
                      n373 = Empty String/Path?(string/path=w978) -> (empty?=w977:bool)
                      n374 = Select(t="0", s=w977, f="1") -> (s? t:f=w979:string)
                    }
                  }
                }
                frame "lLocationFilename" {
                }
                frame "lLocationRotations" {
                  n375 = global read "Results_plotter_Global.vi" "3D Ch Names"() -> (w985:string[])
                  n376 = Index Array(array=w985, index=3) -> (element=w983:string)
                  n377 = Index Array(array=w987, index (col)=2 ("disabled index (col)")) -> (element=w990:string[])  [unwired: 1 in]
                  n378 = Index Array(array=w987, index (col)=0 ("disabled index (col)")) -> (element=w991:string[])  [unwired: 1 in]
                  n379 = Search 1D Array(1D array=w991, element=w983) -> (index of element=w992:i32)  [unwired: 1 in]
                  n380 = Index Array(array=w990, index=w992) -> (element=w994:string)
                  n381 = Fract/Exp String To Number(string=w994, default (0 dbl)=nan ("default (0 DBL)")) -> (number=w996:dbl)  [unwired: 2 in, 1 out]
                  n382 = Negate(x=w996) -> (-x=w997:dbl)
                  n383 = Format Into String(format string="0;0;%.3f", w997) -> (resulting string=w986:string)  [unwired: 2 in, 1 out]
                }
                frame "lRefArrowBaseCoord" {
                }
                frame "lRefArrowColor" {
                }
                frame "lRefArrowComponents" {
                }
                frame "lRefArrowSize" {
                }
                frame "lRefPointColor" {
                }
                frame "lRefPointCoord" {
                }
                frame "lRefPointSize" {
                }
                frame "lViewAngles" {
                }
                frame "mFontSize" {
                }
                frame "mGraphsxColumn" {
                  n384 = Number To Decimal String(number="nCols") -> (decimal integer string=w1008:string)  [unwired: 1 in]
                }
                frame "mGraphsxRow" {
                  n385 = Number To Decimal String(number="nRows") -> (decimal integer string=w1009:string)  [unwired: 1 in]
                }
                frame "mLegendColumnNr" {
                  n386 = local read "No of Series"() -> (w1018:i32)
                  n387 = Divide(x=w1018, y=4) -> (x/y=w1011:dbl)
                  n388 = Round Toward +Infinity(x=w1011) -> (ceil(x): smallest int >= x=w1012:dbl)
                  n389 = Greater?(x=w1011, y=1.0) -> (0:w1016:bool)
                  n390 = To Long Integer(number=w1012) -> (32bit integer=w1015:i32)
                  n391 = Select(t=w1015, s=w1016, f=1) -> (s? t:f=w1013:i32)
                  n392 = Number To Decimal String(number=w1013) -> (decimal integer string=w1019:string)  [unwired: 1 in]
                }
                frame "mLegendLocation" {
                  n393 = local read "Legend Location"() -> (w1021:string)
                }
                frame "mLegendTitle" {
                }
                frame "mMainTitle" {
                  n394 = local read "Final Title"() -> (w1023:string)
                }
                frame "mMainTitleFontSize" {
                }
                frame "pAxisYright" {
                  n395 = Index Array(array=w1025, index=w1031) -> (element=w1030:T2)
                  n396 = Unbundle By Name(w1030) -> ("Right Y?"=w1027:bool)
                  n397 = Select(t="1", s=w1027, f="0") -> (s? t:f=w1026:string)
                }
                frame "pFigureNr" {
                  n398 = Number To Decimal String(number=w1032) -> (decimal integer string=w1033:string)  [unwired: 1 in]
                }
                frame "pFitEquation" {
                  n399 = global read "Results_plotter_Global.vi" "Transpose"() -> (w1034:bool)
                  n400 = case shown="\"Guass glc\"" "Fit type" {
                    tunnel: ["" w1038 w1042 w1046 w1050 w1054 w1058 w1064] -> w1036
                    tunnel: w1034 -> [_ w1041 w1045 w1049 w1053 w1057 w1061 w1065]
                    frame "None" {
                    }
                    frame "Gauss Lat" {
                      n401 = Select(t="C(1)*exp(-((Y-C(2)).^2)/(2*C(3).^2))", s=w1041, f="C(1)*exp(-((X-C(2)).^2)/(2*C(3).^2))") -> (s? t:f=w1038:string)
                    }
                    frame "Gauss Vert" {
                      w1043 = "C(1)*(exp(-((X-C(2)).^2)/(2*C(3).^2))+exp(-((X+C(2)).^2)/(2*C(3).^2)))"  # C(1)*(exp(-((X-C(2)).^2)/(2*C(3).^2))+exp(-((X+C(2)).^2)/(2*C(3).^2)))
                      w1044 = "C(1)*(exp(-((Y-C(2)).^2)/(2*C(3).^2))+exp(-((Y+C(2)).^2)/(2*C(3).^2)))"  # C(1)*(exp(-((Y-C(2)).^2)/(2*C(3).^2))+exp(-((Y+C(2)).^2)/(2*C(3).^2)))
                      n402 = Select(t=w1044, s=w1045, f=w1043) -> (s? t:f=w1042:string)
                    }
                    frame "2nd Poly" {
                      n403 = Select(t="C(1)+C(2)*Y+C(3)*Y.^2", s=w1049, f="C(1)+C(2)*X+C(3)*X.^2") -> (s? t:f=w1046:string)
                    }
                    frame "Linear" {
                      n404 = Select(t="C(1)+C(2)*Y", s=w1053, f="C(1)+C(2)*X") -> (s? t:f=w1050:string)
                    }
                    frame "3rd Poly" {
                      n405 = Select(t="C(1)+C(2)*Y+C(3)*Y.^2+C(4)*Y.^3", s=w1057, f="C(1)+C(2)*X+C(3)*X.^2+C(4)*X.^3") -> (s? t:f=w1054:string)
                    }
                    frame "4th Poly" {
                      n406 = Select(t="C(1)+C(2)*Y+C(3)*Y.^2+C(4)*Y.^3+C(5)*Y.^4", s=w1061, f="C(1)+C(2)*X+C(3)*X.^2+C(4)*X.^3+C(5)*X.^4") -> (s? t:f=w1058:string)
                    }
                    frame "Guass glc" {
                      w1063 = "C(1)*((X/C(2)).^(-(1+C(3))*C(4))*(exp(((1+C(3))/2)*(1-(X/C(2)).^(-2*C(4))))))"  # C(1)*((X/C(2)).^(-(1+C(3))*C(4))*(exp(((1+C(3))/2)*(1-(X/C(2)).^(-2*C(4))))))
                      n407 = Select(t="C(1)*((Y/C(2)).^(-(1+C(3))*C(4))*(exp(((1+C(3))/2)*(1-(Y/C(2)).^(-2*C(4))))))", s=w1065, f=w1063) -> (s? t:f=w1064:string)
                    }
                  }
                }
                frame "pFitIndepAxis" {
                  n408 = global read "Results_plotter_Global.vi" "Transpose"() -> (w1067:bool)
                  n409 = Select(t="Y", s=w1067, f="X") -> (s? t:f=w1066:string)
                }
                frame "pFitIndepAxisFitRange" {
                  n410 = global read "Results_plotter_Global.vi" "Transpose"() -> (w1077:bool)
                  n411 = Index Array(array=w1080, index=w1079) -> (element=w1076:cluster{dbl[], dbl[]})
                  n412 = Unbundle(w1076) -> (w1072:dbl[], w1074:dbl[])
                  n413 = case shown="False" w1077 {
                    tunnel: [w1082 w1084] -> _
                    tunnel: w1074 -> [w1082 w1083]
                    tunnel: [w1081 w1083] -> w1073
                    tunnel: w1072 -> [w1081 w1084]
                    frame False {
                    }
                    frame True {
                    }
                  }
                  n414 = Array Max & Min(array=w1073) -> (max value=w1070:dbl, min value=w1071:dbl)  [unwired: 2 out]
                  n415 = Format Into String(format string="[%f;%f]", w1071, w1070) -> (resulting string=w1078:string)  [unwired: 2 in, 1 out]
                }
                frame "pFitIndepAxisPlotRange" {
                  n416 = global read "Results_plotter_Global.vi" "Transpose"() -> (w1092:bool)
                  n417 = Index Array(array=w1095, index=w1094) -> (element=w1091:cluster{dbl[], dbl[]})
                  n418 = Unbundle(w1091) -> (w1087:dbl[], w1089:dbl[])
                  n419 = case shown="False" w1092 {
                    tunnel: [w1097 w1099] -> _
                    tunnel: w1089 -> [w1097 w1098]
                    tunnel: [w1096 w1098] -> w1088
                    tunnel: w1087 -> [w1096 w1099]
                    frame False {
                    }
                    frame True {
                    }
                  }
                  n420 = Array Max & Min(array=w1088) -> (max value=w1085:dbl, min value=w1086:dbl)  [unwired: 2 out]
                  n421 = Format Into String(format string="[%f;%f]", w1086, w1085) -> (resulting string=w1093:string)  [unwired: 2 in, 1 out]
                }
                frame "pFitLowerBound" {
                  n422 = local read "Fit type"() -> (w1102:T9)
                  n423 = case shown="\"Linear\"" w1102 {
                    tunnel: w1101 -> [_ _ _ _ _ _ _ _]
                    tunnel: ["[6;0;]" ("Legend Location") "0;-inf;0;" ("Legend Location") "0;0;0;" ("Legend Location") "0;0;0;0;" ("Legend Location") "[-inf;-inf;-inf]" ("Legend Location") "[-inf;-inf;-inf;-inf]" ("Legend Location") "[-inf;-inf;-inf;-inf;-inf;]" ("Legend Location") "[-inf;-inf;]" ("Legend Location")] -> w1100
                    frame "None" {
                    }
                    frame "Gauss Lat" {
                    }
                    frame "Gauss Vert" {
                    }
                    frame "Guass glc" {
                    }
                    frame "2nd Poly" {
                    }
                    frame "3rd Poly" {
                    }
                    frame "4th Poly" {
                    }
                    frame "Linear" {
                    }
                  }
                }
                frame "pFitOn" {
                  n424 = Index Array(array=w1114, index=w1116) -> (element=w1115:T2)
                  n425 = Unbundle By Name(w1115) -> ("Fit?"=w1113:bool)
                  n426 = local read "Fit type"() -> (w1111:T9)
                  n427 = case shown="Default" w1111 {
                    tunnel: w1113 -> [_ w1119]
                    tunnel: ["0" ("t") w1118] -> w1112
                    frame "None" {
                    }
                    frame Default {
                      n428 = Select(t="1", s=w1119, f="0") -> (s? t:f=w1118:string)
                    }
                  }
                }
                frame "pFitStart" {
                  n429 = local read "Fit type"() -> (w1126:T9)
                  n430 = global read "Results_plotter_Global.vi" "Transpose"() -> (w1122:bool)
                  n431 = case shown="\"Guass glc\"" w1126 {
                    tunnel: w1125 -> [_ w1145 w1168 _ _ _ _]
                    tunnel: w1124 -> [_ w1144 w1167 _ _ _ _]
                    tunnel: ["[6;0;200]" ("Legend Location") w1133 w1157 "[1;1;1]" ("Legend Location") "[1;1;1;1]" ("Legend Location") "[1;1;1;1;1]" ("Legend Location") "[1;1;]" ("Legend Location")] -> w1123
                    tunnel: w1122 -> [_ w1132 w1156 _ _ _ _]
                    frame "None" {
                    }
                    frame "Gauss Lat", "Gauss Vert" {
                      n432 = Index Array(array=w1145, index=w1144) -> (element=w1143:cluster{dbl[], dbl[]})
                      n433 = Unbundle(w1143) -> (w1128:dbl[], w1130:dbl[])
                      n434 = case shown="False" w1132 {
                        tunnel: [w1147 w1149] -> w1131
                        tunnel: w1130 -> [w1147 w1148]
                        tunnel: [w1146 w1148] -> w1129
                        tunnel: w1128 -> [w1146 w1149]
                        frame False {
                        }
                        frame True {
                        }
                      }
                      n435 = Array Max & Min(array=w1131) -> (max value=w1137:dbl, max index (indices)=w1142:i32)  [unwired: 2 out]
                      n436 = Array Max & Min(array=w1129) -> (max value=w1141:dbl, min value=w1140:dbl)  [unwired: 2 out]
                      n437 = Subtract(x=w1141, y=w1140) -> (x-y=w1139:dbl)
                      n438 = Index Array(array=w1129, index=w1142) -> (element=w1136:dbl)
                      n439 = Divide(x=w1139, y=8.0) -> (x/y=w1135:dbl)
                      n440 = Format Into String(format string="[%f;%f;%f]", w1137, w1136, w1135) -> (resulting string=w1133:string)  [unwired: 2 in, 1 out]
                    }
                    frame "Guass glc" {
                      n441 = Index Array(array=w1168, index=w1167) -> (element=w1166:cluster{dbl[], dbl[]})
                      n442 = Unbundle(w1166) -> (w1152:dbl[], w1154:dbl[])
                      n443 = case shown="False" w1156 {
                        tunnel: [w1170 w1172] -> w1155
                        tunnel: w1154 -> [w1170 w1171]
                        tunnel: [w1169 w1171] -> w1153
                        tunnel: w1152 -> [w1169 w1172]
                        frame False {
                        }
                        frame True {
                        }
                      }
                      n444 = Array Max & Min(array=w1155) -> (max value=w1160:dbl, max index (indices)=w1165:i32)  [unwired: 2 out]
                      n445 = Array Max & Min(array=w1153) -> (max value=w1164:dbl, min value=w1163:dbl)  [unwired: 2 out]
                      n446 = Subtract(x=w1164, y=w1163) -> (x-y=w1162:dbl)
                      n447 = Index Array(array=w1153, index=w1165) -> (element=w1159:dbl)
                      n448 = Divide(x=w1162, y=8.0) -> ()  [unwired: 1 out]
                      n449 = Format Into String(format string="[%f;%f;%f,%f]", w1160, w1159, 1.0 ("input 3"), 0.73 ("input 4")) -> (resulting string=w1157:string)  [unwired: 2 in, 1 out]
                    }
                    frame "2nd Poly" {
                    }
                    frame "3rd Poly" {
                    }
                    frame "4th Poly" {
                    }
                    frame "Linear" {
                    }
                  }
                }
                frame "pLegendLabel" {
                  n450 = local read "Plot Legends Auto"() -> (w1180:string[])
                  n451 = Select(t=w1180, s="Plot Legends", f="Plot Legends Manual") -> (s? t:f=w1179:string[])
                  n452 = Index Array(array=w1179, index=w1177) -> (element=w1178:string)
                }
                frame "pLineColor" {
                  # "pLineColor = {}; %['r','g','b','c','m','y','k','w'] or hexadecimal (e.g. #FF0000)"
                  n453 = Index Array(array=w1183, index=w1186) -> (element=w1185:T2)
                  n454 = Unbundle By Name(w1185) -> ("Color"=w1184:string)
                }
                frame "pLineMarker" {
                  n455 = Index Array(array=w1188, index=w1190) -> (element=w1189:T2)
                  n456 = Unbundle By Name(w1189) -> ("Marker"=w1187:string)
                }
                frame "pLineStyle" {
                  n457 = Index Array(array=w1191, index=w1195) -> (element=w1194:T2)
                  n458 = Unbundle By Name(w1194) -> ("LStyle"=w1193:string)
                  n459 = case shown="\"solid\"" w1193 {
                    selector: w1193 -> [w1196 _]
                    tunnel: [w1196 "-"] -> w1192
                    frame Default {
                    }
                    frame "solid" {
                    }
                  }
                }
                frame "pLineWidth" {
                  n460 = Index Array(array=w1199, index=w1201) -> (element=w1200:T2)
                  n461 = Unbundle By Name(w1200) -> ("LWidth"=w1198:string)
                }
                frame "Plot Index" {
                  n462 = Number To Decimal String(number=w1203) -> (decimal integer string=w1202:string)  [unwired: 1 in]
                }
                frame "pMarkerSize" {
                  n463 = Index Array(array=w1205, index=w1207) -> (element=w1206:T2)
                  n464 = Unbundle By Name(w1206) -> ("Marker size"=w1204:string)
                }
                frame Default {
                }
              }
            }
            n465 = Select(t=w733, s=w740, f=w732) -> (s? t:f=w744:i32)
          }
          n466 = Greater Than 0?(x=w725) -> (x > 0?=w722:bool)
          n467 = Select(t=w716, s=w722, f=w717) -> (s? t:f=w726:i32)
        }
        "Table" <- w705
      }
      frame "Save input file" {
        # "Create matching output directory, as MATLAB won't, and it may not exist, if running from EXE"
        n468 = Index Array(array=w1222, index (col)=0 ("disabled index (col)")) -> (element=w1220:string[])  [unwired: 1 in]
        n469 = local read "Table"() -> (w1219:string[][])
        n470 = Build Array (concatenate)(w1220, w1219) -> (w1218:string[][])
        n471 = Build Path(base path=w1226, name or relative path="Input1D.xls") -> (appended path=w1227:path)
        n472 = Array Subset(array=w1218, index (col)=1 ("index")) -> (w1217:string[][])  [unwired: 3 in]
        n473 = Array To Spreadsheet String(array=w1217, 3:"%s" ("format string")) -> (spreadsheet string=w1228:string)  [unwired: 1 in]
        n474 = Write to Text File(file (use dialog)=w1227, text=w1228) -> (refnum out=w1215:refnum<file>, error out=w1216:errorcluster)  [unwired: 2 in, 1 out]
        n475 = Build Path(base path=w1211, name or relative path="Output") -> (appended path=w1213:path)
        n476 = Close File(refnum=w1215, error in=w1216) -> (error out=w1214:errorcluster)  [unwired: 1 out]
        n477 = Build Path(base path=w1213, name or relative path=w1210) -> (appended path=w1209:path)
        n478 = call <vilib>:"Create Directory Recursive.vi"("error in (no error)"=w1214, "directory"=w1209) -> ()  [unwired: 3 in, 3 out]
      }
      frame "Run MATLAB Code" {
        n479 = call "Call_MATLAB_Suite.vi"("Mode"=MATLAB_Mode."1D Plotter") -> ("Output file"=→"Output file":path, "error out"=w1232:errorcluster)  [unwired: 2 in, 1 out]
        n480 = case shown="Error .." w1232 {
          selector: w1232 -> [_ w1243]
          tunnel: [TRUE ("f") FALSE ("f")] -> w1239
          frame No Error {
          }
          frame Error {
            n481 = Unbundle By Name(w1243) -> ("source"=w1242:string)
            n482 = One Button Dialog(message=w1242) -> ()  [unwired: 1 in, 1 out]
          }
        }
        n483 = Select(t="Display PDF with save option", s="Show Save Option?", f="Display PDF" ("t")) -> (s? t:f=w1233:string)
      }
      frame "Display PDF" {
        n484 = local read "Output file"() -> (w1245:path)
        n485 = call "Open PDF in desired reader.vi"("Path"=w1245) -> ()  [unwired: 2 in, 1 out]
      }
      frame "Display PDF with save option" {
        n486 = local read "Output file"() -> (w1251:path)
        n487 = stacked-sequence {
          tunnel: w1251 -> [w1257 w1277]
          tunnel: [w1253 _] -> w1249
          frame #0 {
            n488 = local read "Plot Folder"() -> (w1254:string[])
            n489 = call "Display PDF File for Preview.vi"("Data Directories"=w1254, "PDF file"=w1257) -> ("Filename Out"=w1256:string)  [unwired: 8 in, 1 out]
            n490 = Empty String/Path?(string/path=w1256) -> (empty?=w1255:bool)
            n491 = case shown="False" w1255 {
              tunnel: w1257 -> [w1266 _]
              tunnel: w1256 -> [w1265 _]
              tunnel: w1254 -> [w1264 _]
              tunnel: [w1258 FALSE] -> w1253
              frame False {
                n492 = local read "Duplicate Plot"() -> (w1267:bool)
                n493 = global read "Results_plotter_Global.vi" "Template"() -> (w1262:path)
                n494 = call "Save PDF files.vi"("Duplicate Plot"=w1267, "Open in Acrobat"="Open in Acrobat", "Desired Filename"=w1265, "Data Directories"=w1264, "PDF file in"=w1266) -> ("Saved Files"=→"Saved Files":path[], "Results Folders"=w1263:path[])  [unwired: 5 in]
                n495 = local read "Fit type"() -> (w1259:T9)
                n496 = Strip Path(path=w1262) -> (name=w1261:string)  [unwired: 1 out]
                n497 = for {
                  tunnel: w1263 -> [w1275] mode=indexing
                  tunnel: w1262 -> [w1274]
                  tunnel: w1261 -> [w1272]
                  n498 = Strip Path(path=w1275) -> (stripped path=w1273:path)  [unwired: 1 out]
                  n499 = Build Path(base path=w1273, name or relative path=w1272) -> (appended path=w1271:path)
                  n500 = Copy(10:w1271, 11:w1274) -> ()  [unwired: 3 in, 3 out]
                }
                n501 = case shown="\"None\"" w1259 {
                  tunnel: [FALSE TRUE] -> w1258
                  frame "None" {
                  }
                  frame Default {
                  }
                }
                n502 = call "Save Plotted Data File Rows.vi"("Results Folders"=w1263) -> ()  [unwired: 5 in]
              }
              frame True {
              }
            }
          }
          frame #1 {
            n503 = Delete(path (use dialog)=w1277) -> ()  [unwired: 4 in, 3 out]
          }
        }
      }
      frame "Get Fit Coeff" {
        n504 = stacked-sequence {
          seq-local: [w1287 _ _] -> [_ w1331 _]
          seq-local: [w1305 _ _] -> [_ w1337 _]
          seq-local: [_ w1330 _] -> [_ _ w1405]
          seq-local: [_ w1329 _] -> [_ _ w1402]
          seq-local: [_ w1328 _] -> [_ _ w1400]
          tunnel: w1279 -> [w1312 _ _]
          tunnel: w1278 -> [_ w1334 _]
          frame #0 {
            w1289 = "pFitEquation"
            n505 = Index Array(array=w1312, index (col)=0 ("disabled index (col)")) -> (element=w1304:string[])  [unwired: 1 in]
            n506 = global read "Constants_global.vi" "MATLAB Folder"() -> (w1298:path)
            n507 = local read "Table"() -> (w1303:string[][])
            n508 = Search 1D Array(1D array=w1304, element="pFitOn") -> (index of element=w1309:i32)  [unwired: 1 in]
            n509 = Search 1D Array(1D array=w1304, element=w1289) -> (index of element=w1302:i32)  [unwired: 1 in]
            n510 = Build Path(base path=w1298, name or relative path="Output") -> (appended path=w1301:path)
            n511 = Index Array(array=w1303, index (col)=w1309) -> (element=→"subarray":string[])  [unwired: 1 in]
            n512 = Index Array(array=w1303, index (col)=w1302) -> (element=w1290:string[])  [unwired: 1 in]
            n513 = Index Array(array=w1303, index (col)=0 ("disabled index (col)")) -> (element=w1306:string[])  [unwired: 1 in]
            n514 = Build Path(base path=w1301, name or relative path="1D") -> (appended path=w1296:path)
            n515 = Build Array (concatenate)(w1289, w1290) -> (w1288:string[])
            n516 = Decimal String To Number(string=w1306) -> (number=w1305:i32[])  [unwired: 2 in, 1 out]
            n517 = Build Path(base path=w1296, name or relative path="FittingCoefficients.xls") -> (appended path=w1295:path)
            n518 = local read "Fit type"() -> (w1286:T9)
            n519 = Read from Text File(file (use dialog)=w1295) -> (text=w1294:string)  [unwired: 3 in, 3 out]
            n520 = Spreadsheet String To Array(format string="%s", spreadsheet string=w1294, array type (2D Dbl)=string[][] []) -> (array=w1285:string[][])  [unwired: 1 in]
            n521 = for {
              tunnel: w1288 -> [w1320] mode=indexing
              tunnel: [w1319] -> w1284 mode=indexing
              tunnel: w1286 -> [w1318]
              tunnel: w1285 -> [w1317] mode=indexing
              n522 = case shown="\"Gauss Lat\", \"Gauss Vert\"" w1318 {
                tunnel: [0 3 4 2 3 4 5] -> w1314
                frame "None" {
                }
                frame "Gauss Lat", "Gauss Vert" {
                }
                frame "Guass glc" {
                }
                frame "Linear" {
                }
                frame "2nd Poly" {
                }
                frame "3rd Poly" {
                }
                frame "4th Poly" {
                }
              }
              n523 = Add(x=w1314, y=3) -> (x+y=w1316:i32)
              n524 = Array Subset(array=w1317, length=w1316) -> (w1313:string[])  [unwired: 1 in]
              n525 = Build Array (concatenate)(w1313, w1320) -> (w1319:string[])
            }
            "Coeff" <- w1284
            n526 = Array Subset(array=w1284, index (row)=1 ("index"), index (col)=2 ("index")) -> (w1287:string[][])  [unwired: 2 in]
          }
          frame #1 {
            n527 = call "Fast_string_Replace.vi"("Replace match with:"="", "Input String"=w1334, "matchThis"=":" ("regular expression")) -> ("Output String"=w1333:string)  [unwired: 1 in, 1 out]
            n528 = global read "Results_plotter_Global.vi" "Plot Metadata"() -> (w1338:T12[])
            n529 = local read "Fit type"() -> (w1332:T9)
            n530 = for {
              tunnel: w1338 -> [w1349]
              tunnel: w1337 -> [w1347] mode=indexing
              tunnel: w1333 -> [w1345]
              tunnel: w1332 -> [w1344]
              tunnel: [w1343] -> w1330
              tunnel: [w1342] -> w1328 mode=concatenating
              tunnel: w1331 -> [w1340] mode=indexing
              tunnel: [w1339] -> w1329 mode=concatenating
              n531 = case shown="\"Guass glc\"" w1344 {
                tunnel: [string[] [] w1357 w1362 w1369 w1377 w1385 w1387 w1396] -> w1346
                frame "None" {
                }
                frame "Linear" {
                  n532 = Build Array(":Offset:A", ":Grad:B", ":Fit:Error", ":FitFormula:") -> (w1357:string[])
                }
                frame "2nd Poly" {
                  n533 = Build Array(":Coeff:A", ":Coeff:B", ":Coeff:C", ":Fit:Error", ":FitFormula:") -> (w1362:string[])
                }
                frame "3rd Poly" {
                  n534 = Build Array(":Coeff:A", ":Coeff:B", ":Coeff:C", ":Coeff:D", ":Fit:Error", ":FitFormula:") -> (w1369:string[])
                }
                frame "4th Poly" {
                  n535 = Build Array(":Coeff:A", ":Coeff:B", ":Coeff:C", ":Coeff:D", ":Coeff:E", ":Fit:Error", ":FitFormula:") -> (w1377:string[])
                }
                frame "Gauss Lat" {
                  n536 = Build Array(":Max:Lat", ":Yo:", ":Sig Y:", ":Fit:Error", ":FitFormula:") -> (w1385:string[])
                }
                frame "Gauss Vert" {
                  n537 = Build Array(":Max:Vert", ":Zp:", ":Sig Z:", ":Fit:Error", ":FitFormula:") -> (w1387:string[])
                }
                frame "Guass glc" {
                  n538 = Build Array(":MaxC:glc", ":MaxX:glc", ":m:glc", ":q:glc", ":Fit:Error", ":FitFormula:") -> (w1396:string[])
                }
              }
              n539 = Index Array(array=w1349, index=w1347) -> (element=w1348:T12)
              n540 = Unbundle By Name(w1348) -> ("Row Number"=w1342:i32[])
              n541 = for {
                tunnel: w1345 -> [w1353]
                tunnel: w1346 -> [w1352] mode=indexing
                tunnel: [w1351] -> w1343 mode=indexing
                n542 = Concatenate Strings(w1353, w1352) -> (w1351:string)
              }
              n543 = Array Size(array=w1342) -> (size(s)=w1341:i32)
              n544 = for {
                N: w1341 -> [_]
                tunnel: w1340 -> [w1350]
                tunnel: [w1350] -> w1339 mode=indexing
              }
            }
          }
          frame #2 {
            n545 = case shown="True" "Put Coeff\nin Results file" {
              tunnel: w1405 -> [_ w1412]
              tunnel: [string[] [] w1412] -> w1404
              tunnel: [string[][] [] w1411] -> w1403
              tunnel: w1402 -> [_ w1411]
              tunnel: [i32[] [] ("Row Number") w1410] -> w1401
              tunnel: w1400 -> [_ w1410]
              frame False {
              }
              frame True {
              }
            }
            n546 = global write "Results_plotter_Global.vi" "New Chs In"(w1404) -> ()
            n547 = global write "Results_plotter_Global.vi" "New Values In"(w1403) -> ()
            n548 = global write "Results_plotter_Global.vi" "New Values Row index"(w1401) -> ()
          }
        }
      }
      frame "End" {
      }
    }
  }
  "AuditTrail" <- w11
  "Saved Automatically?" <- FALSE
